vi "AutomatedTransfer_v2.vi"() -> ()   [LabVIEW 2013]
uses:
  controls/Control Configuration.ctl
  controls/Digital Controller.ctl
  controls/Motion Observer.ctl
  controls/UI Data.ctl
  controls/All FPGA Configuration Values.ctl
  controls/FPGA State.ctl
  controls/Raw Values.ctl
  Globals/Global - All UI Loop Stop.vi
  Globals/Global - UI Stream and Variable Connections.vi
  Globals/Global - Configuration Options.vi
  support/User Event - Stop/User Event - Stop.lvlib
  support/Message Queue/Message Queue.lvlib
  <vilib>/Analysis/NI_AALBase.lvlib
panel:
  in  "Switch to Safe State":bool
  in  "Exit":bool
  out "System Status":string="\n8/4/2014 6:26:47 PM: RT Error 91 - Variant To Data in RT Main.vi\n8/4/2014 6:26:32 PM: RT Error 91 - Variant To Data in RT Main.vi\n8/4/2014 6:26:21 PM: RT Error 91 - Variant To Data in RT Main.vi\n8/4/2014 6:26:03 PM: RT Error 91 - Variant To Data in RT Main.vi\n8/4/2014 6:25:47 PM: RT Error 91 - Variant To Data in RT Main.vi\n8/4/2014 6:25:36 PM: RT Error 91 - Variant To Data in RT Main.vi\n6/10/2014 3:19:43 PM: UI Error -1950679035 - Read Variable in AutomatedTransfer_v2.vi\n5/12/2014 3:31:58 PM: UI Error -314220 - Read Single Element from Stream in UI - Read Stream from RT.vi->UI Main.vi\n5/12/2014 3:31:58 PM: UI Error -314220 - Read Single Element from Stream in UI - Read Stream from RT.vi->UI Main.vi\n5/12/2014 3:31:58 PM: UI Error -314220 - Read Single Element from Stream in UI - Read Stream from RT.vi->UI Main.vi\n5/12/2014 3:31:58 PM: UI Error -314220 - Read Single Element from Stream in UI - Read Stream from RT.vi->UI Main.vi\n5/12/2014 3:31:58 PM: UI Error -314220 - Read Single Element from Stream in UI - Read Stream from RT.vi->UI Main.vi\n5/12/2014 3:31:58 PM: UI Error -314220 - Read Single Element from Stream in UI - Read Stream from RT.vi->UI Main.vi\n5/12/2014 3:31:58 PM: UI Error -314220 - Read Single Element from Stream in UI - Read Stream from RT.vi->UI Main.vi\n5/12/2014 3:31:58 PM: UI Error -314220 - Read Single Element from Stream in UI - Read Stream from RT.vi->UI Main.vi\n5/12/2014 3:31:58 PM: UI Error -314220 - Read Single Element from Stream in UI - Read Stream from RT.vi->UI Main.vi\n5/12/2014 3:31:58 PM: UI Error -314220 - Read Single Element from Stream in UI - Read Stream from RT.vi->UI Main.vi\n5/12/2014 3:31:58 PM: UI Error -314220 - Read Single Element from Stream in UI - Read Stream from RT.vi->UI Main.vi\n5/12/2014 3:31:58 PM: UI Error -314220 - Read Single Element from Stream in UI - Read Stream from RT.vi->UI Main.vi\n5/12/2014 3:31:58 PM: UI Error -314220 - Read Single Element from Stream in UI - Read Stream from RT.vi->UI Main.vi\n5/12/2014 3:31:58 PM: UI Error -314220 - Read Single Element from Stream in UI - Read Stream from RT.vi->UI Main.vi\n5/12/2014 3:31:58 PM: UI Error -314220 - Read Single Element from Stream in UI - Read Stream from RT.vi->UI Main.vi\n5/12/2014 3:31:58 PM: UI Error -314220 - Read Single Element from Stream in UI - Read Stream from RT.vi->UI Main.vi\n5/12/2014 3:31:58 PM: UI Error -314220 - Write Single Element to Stream in UI Main.vi\n5/12/2014 3:31:36 PM: UI Error -314004 - Create Network Stream Writer Endpoint in UI - Initiate Connection.vi->UI Main.vi\n5/6/2014 11:02:04 PM: UI Error -314220 - Write Single Element to Stream in UI Main.vi"
  out "Current FPGA Control Mode":u16(ring) items=["Safe State", "Manual", "Control (PID)"]
  in  "Settings Tab":T1(tab)
  out "Stage stop position (mm):":dbl=99.99983984375 format="%#.2g"
  out "Test LED":bool
  out "Roller LED":bool=TRUE
  in  "Test control":bool
  in  "Disable test control":bool
  in  "Stage speed (mm/s):":dbl=21.0 min=0.2 max=21.0
  out "Force results (N)":cluster{dbl[], dbl[]}(graph)
  in  "Save Results":bool
  in  "Stop Test":bool
  in  "Run Test":bool
  in  "Stop dwell time (s):":dbl=2.0 min=0.0
  in  "Start dwell time (s):":dbl=2.0 min=0.0
  in  "Travel distance (mm):":dbl=50.0 min=-150.0 max=150.0 step=0.1
  in  "Contact force (N):":fxp<+/-,20,7>=4.0
  out "Measured contact force (N):":dbl
  out "Stage position (mm):":dbl format="%#.2g"
  out "Fthresh (N):":fxp<+/-,16,8>=2.0 format="%.3g"
  in  "Home position (mm)":dbl=3.5
  in  "Stop roller":bool
  in  "Speed (mm/s):":dbl=2.0 min=0.2 max=5.0
  in  "Contact roller":bool
  in  "Disable roller control":bool
  in  "Roller control":bool
  in  "Home Roller":bool
  in  "Auto tare":bool=TRUE
  out "Position (mm):":dbl
  out "Force (N):":dbl
  out "Max speed (mm/s):":dbl=21.0
  out "Max position (mm):":dbl=151.49760546875
  in  "Position (mm):":dbl=85.0 min=0.0 max=150.0 step=0.1
  in  "Stage speed (mm/s):":dbl=21.0 min=0.2 max=21.0
  out "Stage position (mm):":dbl=99.9996015625 format="%#.2g"
  in  "Go stage":bool
  in  "Stop stage":bool
  in  "Home stage":bool
  out "path":path
  in  "Motion Observer":T2
  in  "Control period (ticks)":u32=40000
  in  "Find tare offset":bool=TRUE
  in  "Channel 3 Setpoint":fxp<+/-,16,5>
  in  "Channel 2 Setpoint":fxp<+/-,16,5>
  in  "Channel 1 Setpoint":fxp<+/-,20,7>=24.0
  in  "Channel 0 Setpoint":fxp<+/-,20,7>=4.0
  in  "Update Control Configuration":bool
  in  "Control Configurations":T3[](array[typedef])=[{"PID Gains"={"proportional gain (Kc)"=55.0, "integral gain (Kc*Ts/Ti)"=0.0, "derivative gain (Kc*Td/Ts)"=0.0}, "Output Range"={"output high"=50.0, "output low"=-50.0}}, {"PID Gains"={"proportional gain (Kc)"=0.0, "integral gain (Kc*Ts/Ti)"=0.0, "derivative gain (Kc*Td/Ts)"=0.0}, "Output Range"={"output high"=10.0, "output low"=-10.0}}, {"PID Gains"={"proportional gain (Kc)"=0.0, "integral gain (Kc*Ts/Ti)"=0.0, "derivative gain (Kc*Td/Ts)"=0.0}, "Output Range"={"output high"=10.0, "output low"=-10.0}}, {"PID Gains"={"proportional gain (Kc)"=0.0, "integral gain (Kc*Ts/Ti)"=0.0, "derivative gain (Kc*Td/Ts)"=0.0}, "Output Range"={"output high"=10.0, "output low"=-10.0}}]
  in  "Run Control":bool
  in  "Stop Control":bool
  in  "Digital Controller":T4
  out "Offset (N)":fxp<+/-,16,8>=0.16796875
  in  "Channel 3 Manual Value":fxp<+/-,16,5>
  in  "Channel 2 Manual Value":fxp<+/-,16,5>
  in  "Channel 1 Manual Value":fxp<+/-,16,5>
  in  "Channel 0 Manual Value":fxp<+/-,16,5>
  in  "Run Manual":bool
  in  "Stop Manual":bool
  in  "Retain data":bool
  out "F std":dbl=0.005665196330386121 format="%#_4g"
  out "F avg":dbl=-0.0348828125 format="%#_4g"
  in  "Clear Button":bool
  in  "Pause Button":bool
  in  "Save As Button":bool
  in  "Display frequency (Hz)":dbl=100.0 min=1.0 step=1.0
  out "Inputs (mV or V)":cluster{dbl[], dbl[]}[](graph)
  in  "Number of points":i32=500 min=1 max=999999999
  out "Force (N)":cluster{dbl[], dbl[]}(graph)
  out "V*":cluster{dbl[], dbl[]}(graph)
  out "Roller position (mm)":cluster{dbl[], dbl[]}(graph)
  out "Control loop frequency (Hz)":u32=4294967295
  out "Stage position (mm)":cluster{dbl[], dbl[]}(graph)
  out "Actual Loop Period (ticks)":u32
  out "Largest Contiguous Memory (bytes)":dbl(graph)
  out "CPU Usage (%)":dbl(graph)
  out "Connected?":bool=TRUE
  in  "Connect to Controller":bool
  in  "Controller Address":string="169.254.66.100"
  # "LabVIEW FPGA Control on CompactRIO"
  # "Connection Settings"
  # "Roller panel"
  # "Stage panel"
  # "To do: \n-Wire appropriate connections into R2R-Controller\n-Update Monitoring Loop Rate by changing Display Rate \n  Note: with 1 ms rate, the program hangs\n-Clean up noise in load cell when V* acts"
  # "Warning: Home cannot be stopped"
  # "Test panel"
  # "Force Command (N)"
  # "Position Command (mm)"
  # "Current Command (Testing)"
  # "Control period and setpoint changes are sent to the target automatically."
  # "Control Configuration changes are sent to the target when you click \"Update Control Configurations\"."
  # "Not used"
  # "Not used"
  # "Not used"
  # "F ="
  # "+/-"
  # "N"
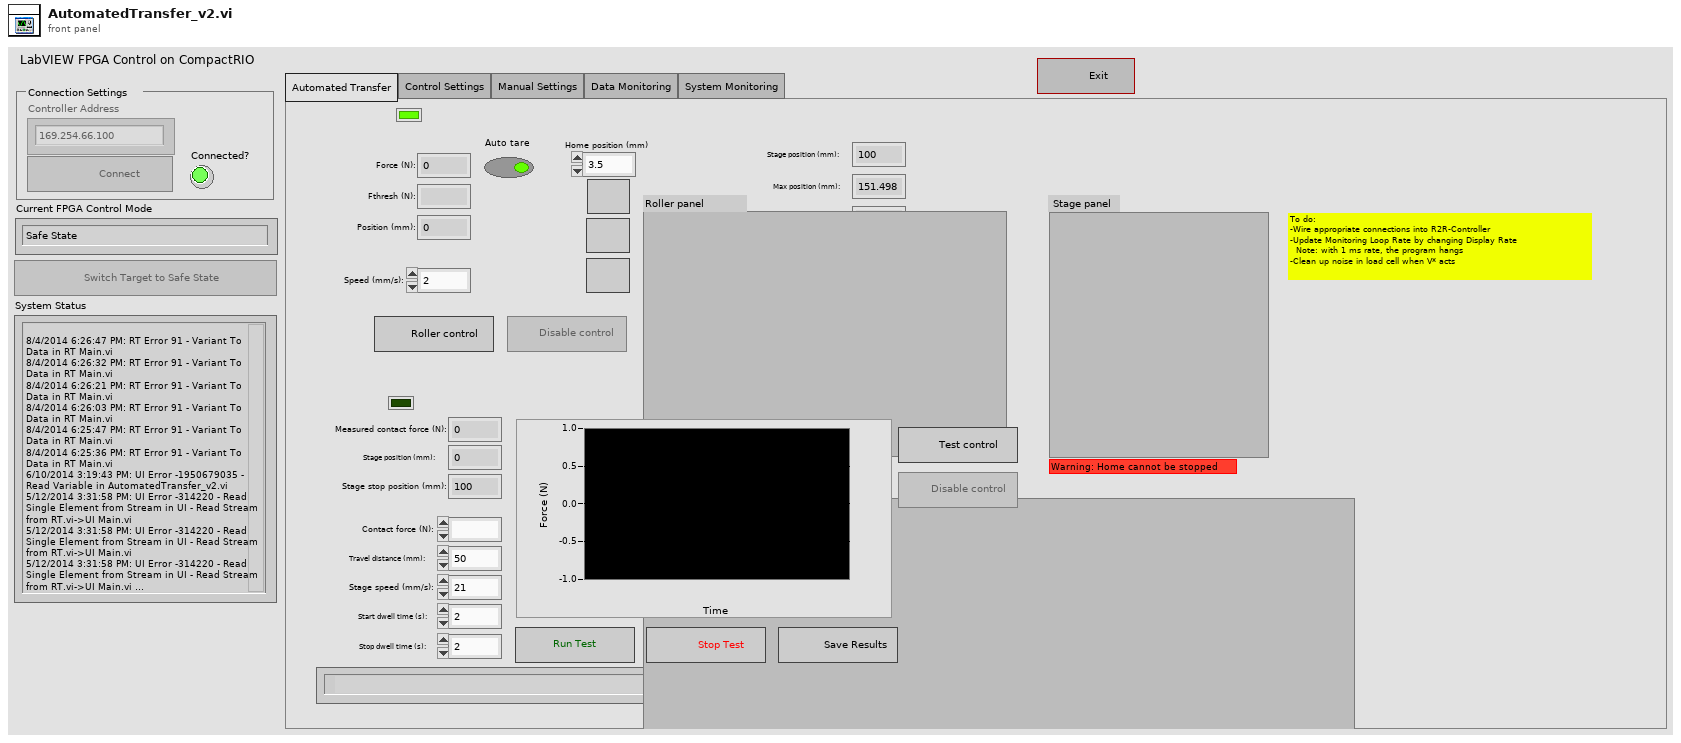
[diagram p1: front panel]
types:
  T1 = enum32{"Automated Transfer", "Control Settings", "Manual Settings", "Data Monitoring", "System Monitoring"}
  T2 = typedef "Motion Observer.ctl" = cluster{"bo (kg/s)":fxp<+/-,20,7>, "kso (N/m)":fxp<+/-,20,7>, "kiso (N/m)":fxp<+/-,20,7>}
  T3 = typedef "Control Configuration.ctl" = cluster{"PID Gains":cluster{"proportional gain (Kc)":fxp<+/-,16,8>, "integral gain (Kc*Ts/Ti)":fxp<+/-,16,8>, "derivative gain (Kc*Td/Ts)":fxp<+/-,16,8>}, "Output Range":cluster{"output high":fxp<+/-,16,7>, "output low":fxp<+/-,16,7>}}
  T4 = typedef "Digital Controller.ctl" = cluster{"kvc (N/m)":fxp<+,16,12>, "ymod (-)":fxp<+/-,16,5>, "Mar (kg)":fxp<+/-,16,8>, "Foff (N)":fxp<+/-,16,8>, "Fthresh (N)":fxp<+/-,16,5>, "ba (kg/s)":fxp<+/-,16,5>, "ksa (N/m)":fxp<+/-,16,5>, "kisa (N/m)":fxp<+/-,16,5>, "k_backemf":fxp<+/-,16,5>, "Frr (N/s)":fxp<+/-,16,5>, "xrr (mm/s)":fxp<+/-,16,5>, "bp (kg/s)":fxp<+/-,16,5>, "k_1 (1/s)":fxp<+/-,16,5>, "k_2 (1/s)":fxp<+/-,16,5>}
  T5 = typedef "UI Data.ctl" = cluster{"Switch to Safe State Ref":refnum<vi>, "Run Manual Ref":refnum<vi>, "Stop Manual Ref":refnum<vi>, "Run Control Ref":refnum<vi>, "Stop Control Ref":refnum<vi>, "Update Control Configurations Ref":refnum<vi>, "Ch 0 Setpoint Ref":refnum<vi>, "Ch 1 Setpoint Ref":refnum<vi>, "Ch 2 Setpoint Ref":refnum<vi>, "Ch 3 Setpoint Ref":refnum<vi>, "Ch 0 Manual Ref":refnum<vi>, "Ch 1 Manual Ref":refnum<vi>, "Ch 2 Manual Ref":refnum<vi>, "Ch 3 Manual Ref":refnum<vi>, "Control Configurations Ref":refnum<vi>, "Control period (ticks) Ref":refnum<vi>, "Roller control":refnum<vi>, "Disable roller control":refnum<vi>, "Test control":refnum<vi>, "Disable test control":refnum<vi>, "Motion Observer":refnum<vi>, "Digital Controller":refnum<vi>}
  T6 = typedef "Message Queue.lvlib/All Message Queues.ctl" = cluster{"UI":refnum<queue>}
  T7 = enum16{"open", "replace", "create", "open or create", "replace or create", "replace or create with confirmation"}
  T8 = cluster{"Channel 0 Setpoint":fxp<+/-,20,7>, "Channel 1 Setpoint":fxp<+/-,20,7>, "Channel 2 Setpoint":fxp<+/-,16,5>, "Channel 3 Setpoint":fxp<+/-,16,5>}
  T9 = cluster{"Channel 0 Manual Value":fxp<+/-,16,5>, "Channel 1 Manual Value":fxp<+/-,16,5>, "Channel 2 Manual Value":fxp<+/-,16,5>, "Channel 3 Manual Value":fxp<+/-,16,5>}
  T10 = typedef "Variable References.ctl" = cluster{"CPU Usage":refnum<k21>, "Contiguous Memory":refnum<k21>, "Input Values":refnum<k21>, "Output Values":refnum<k21>, "FPGA Mode":refnum<k21>, "Actual Loop Period":refnum<k21>}
  T11 = typedef "Raw Values.ctl" = cluster{"Channel 0":fxp<+/-,20,7>, "Channel 1":fxp<+/-,20,7>, "Channel 2":fxp<+/-,20,7>, "Channel 3":fxp<+/-,20,14>}
  T12 = cluster{"Channel 0":dbl, "Channel 1":dbl, "Channel 2":dbl, "Channel 3":dbl}
  T13 = cluster{fxp<+/-,16,5>, "Channel 1 Manual Value":fxp<+/-,16,5>, "Channel 2 Manual Value":fxp<+/-,16,5>, "Channel 3 Manual Value":fxp<+/-,16,5>}
  T14 = cluster{"fixed-point type":fxp<+/-,16,5>, "Channel 1 Manual Value":fxp<+/-,16,5>, "Channel 2 Manual Value":fxp<+/-,16,5>, "Channel 3 Manual Value":fxp<+/-,16,5>}
  T15 = cluster{"Contact force (N): ":fxp<+/-,20,7>, "Channel 1 Setpoint":fxp<+/-,20,7>, "Channel 2 Setpoint":fxp<+/-,16,5>, "Channel 3 Setpoint":fxp<+/-,16,5>}
  T16 = cluster{"Message":string, "Message Data":variant}
  T17 = typedef "All FPGA Configuration Values.ctl" = cluster{"FPGA State":T18, "Manual Values":T11, "Setpoints":T11, "Control Configurations":T3[]}
  T18 = typedef "FPGA State.ctl" = enum16{"Safe State", "Manual", "Control (PID)"}
  T19 = cluster{"Digital Controller":T4, "Motion Observer":T2}
  T20 = cluster{string, cluster{"Digital Controller":T4, "Motion Observer":T2}}
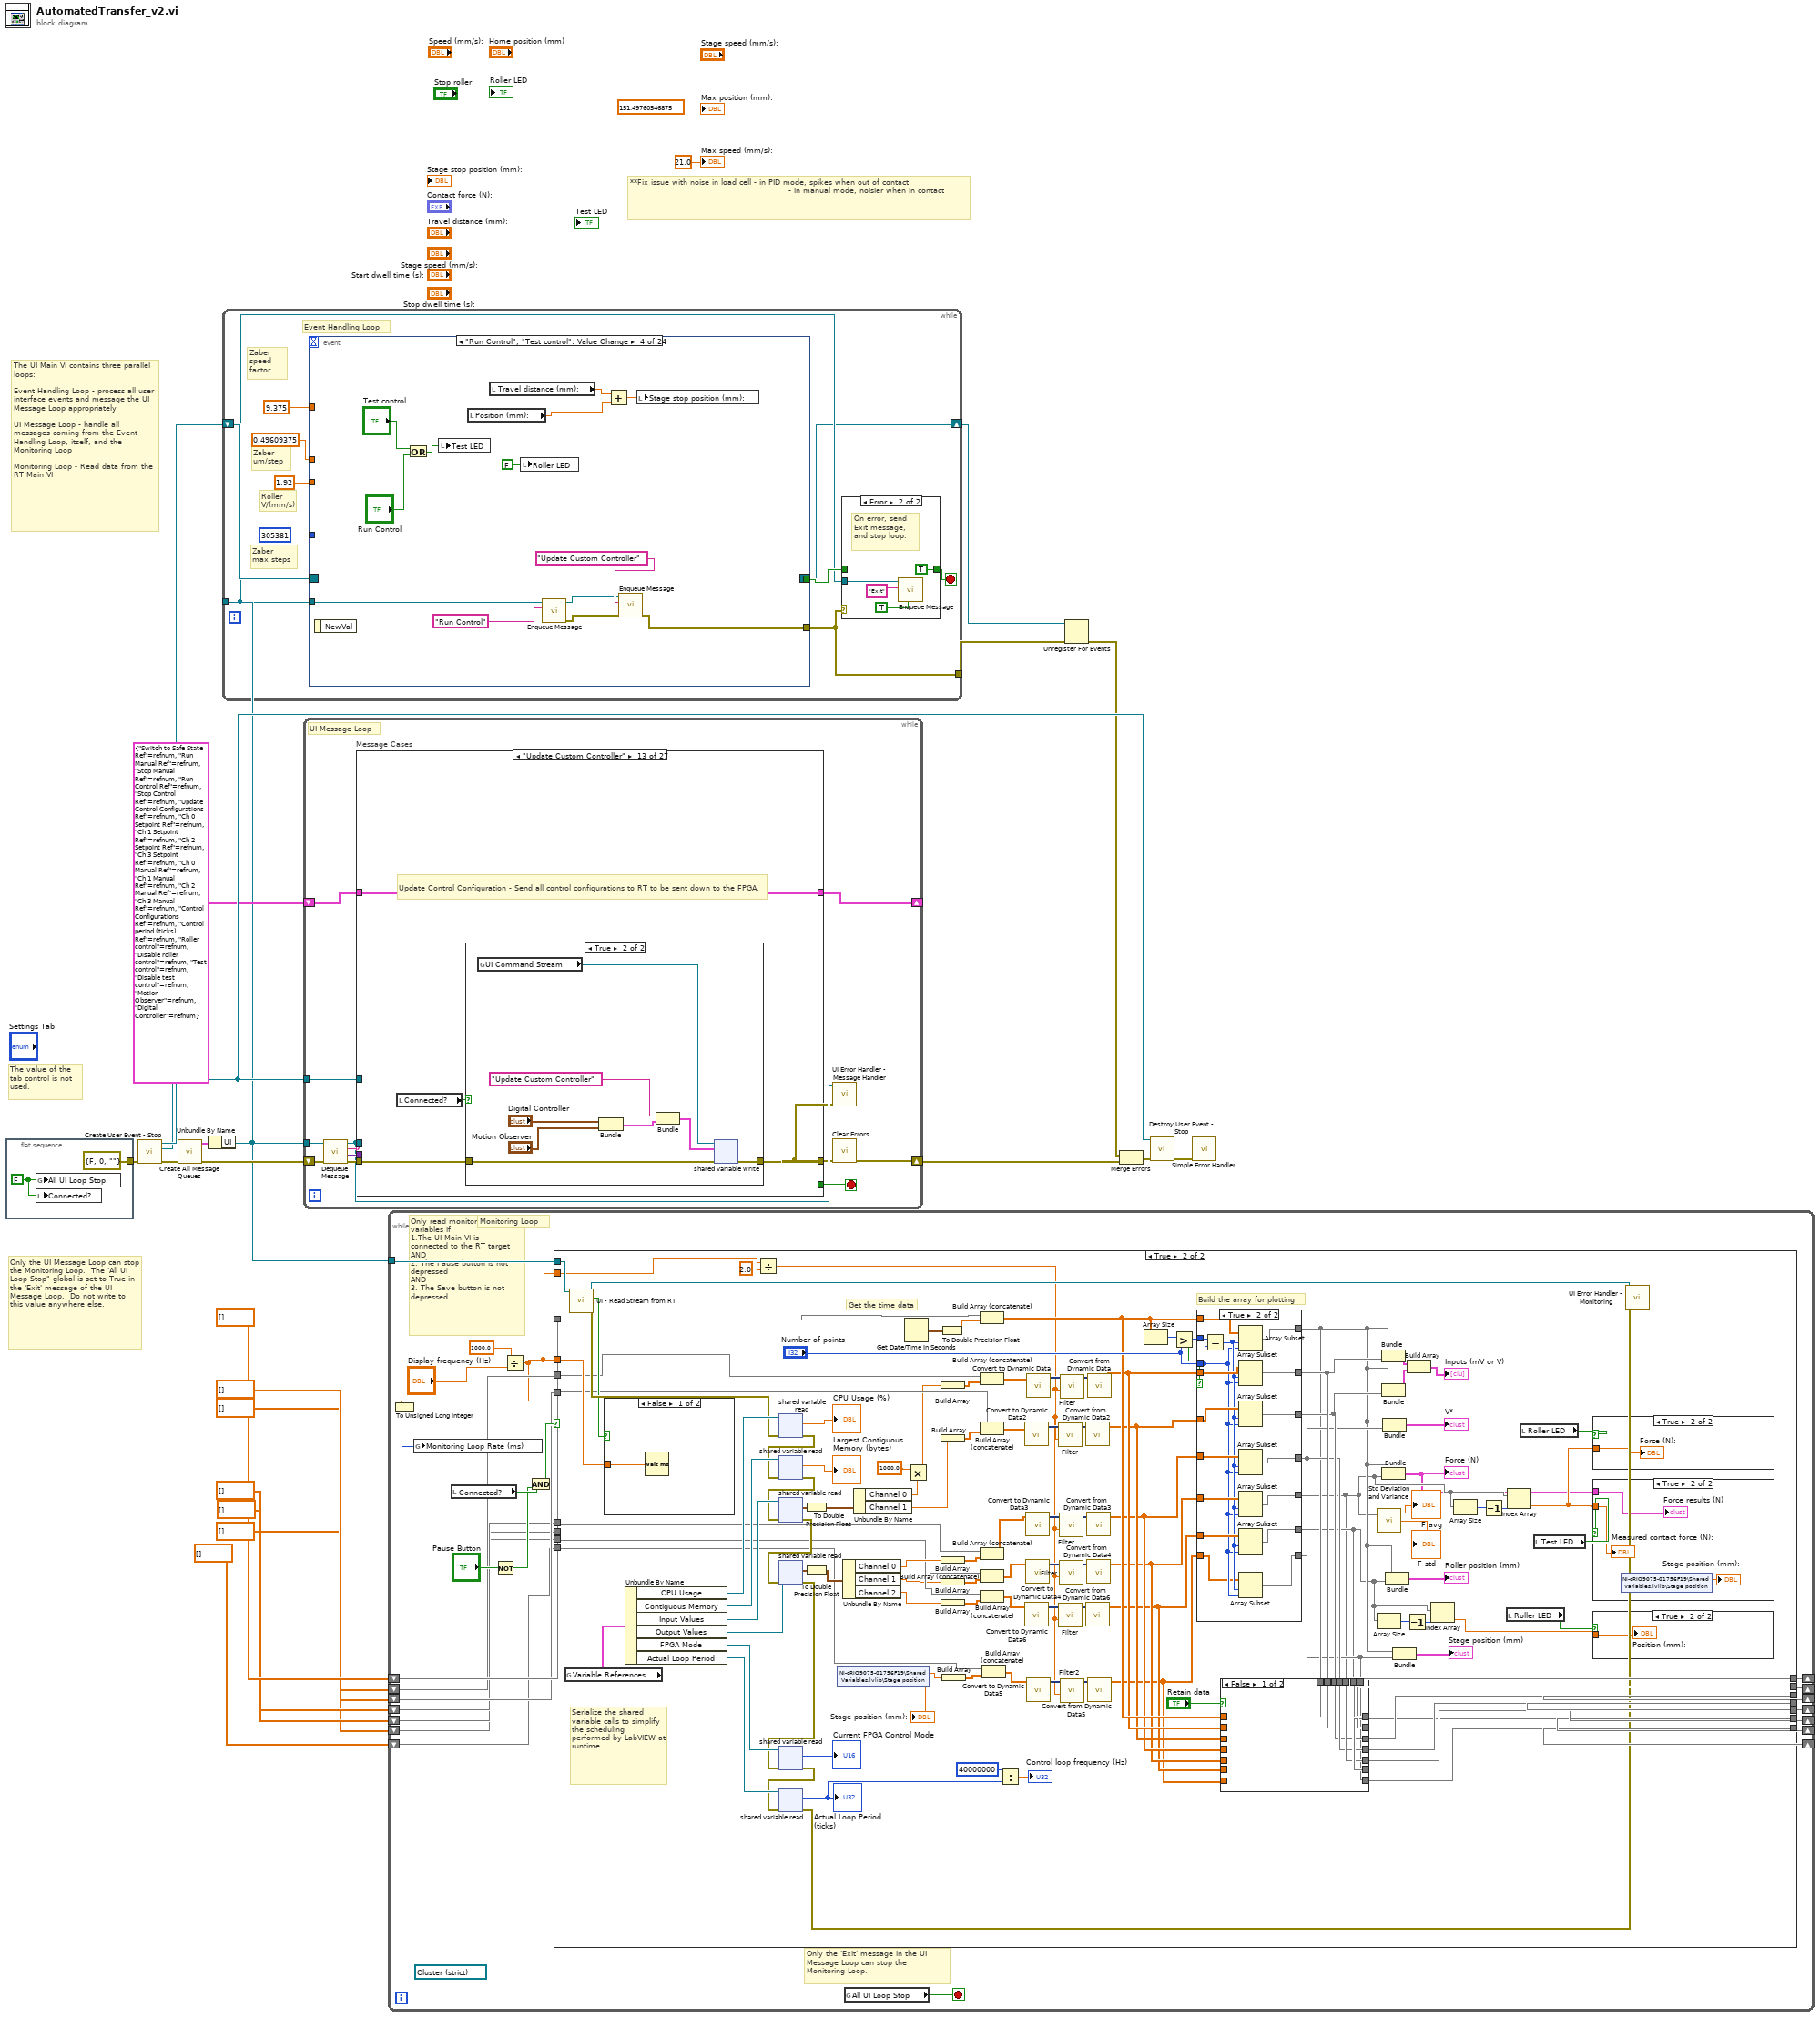
[diagram p0: block diagram]
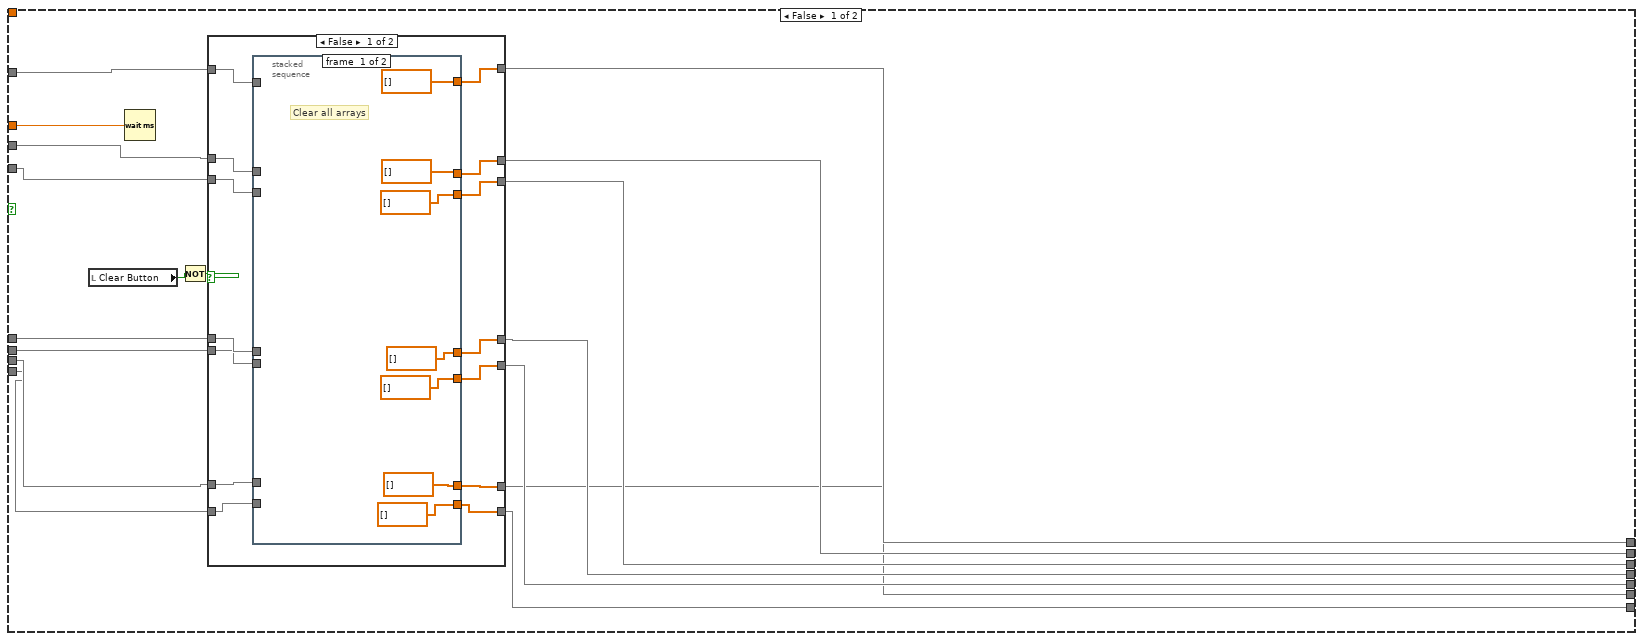
[diagram p2: hidden frame]
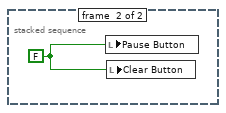
[diagram p3: hidden frame]
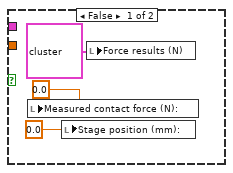
[diagram p5: hidden frame]
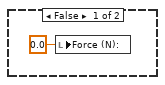
[diagram p6: hidden frame]
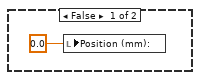
[diagram p7: hidden frame]
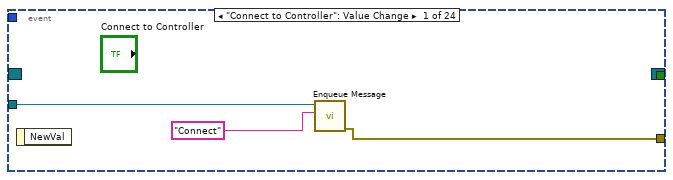
[diagram p12: hidden frame]
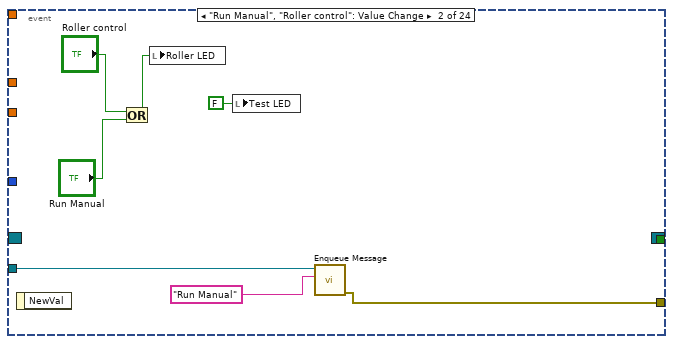
[diagram p13: hidden frame]
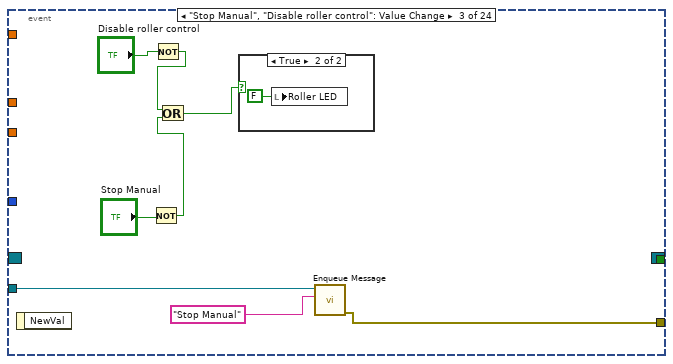
[diagram p14: hidden frame]
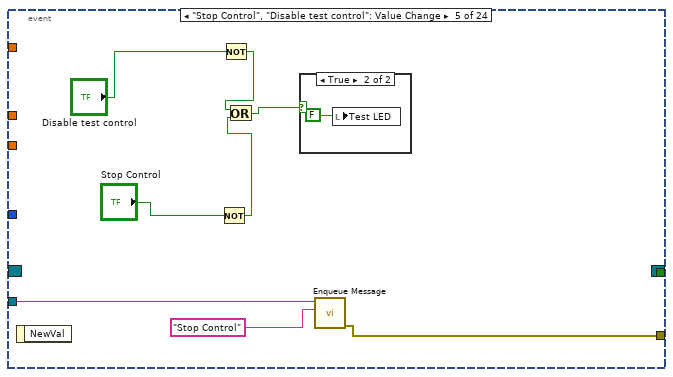
[diagram p16: hidden frame]
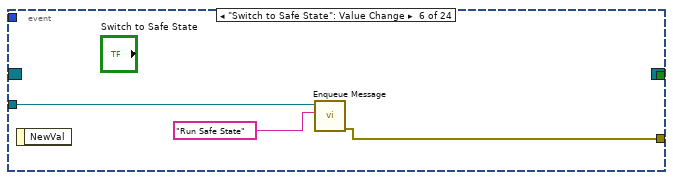
[diagram p18: hidden frame]
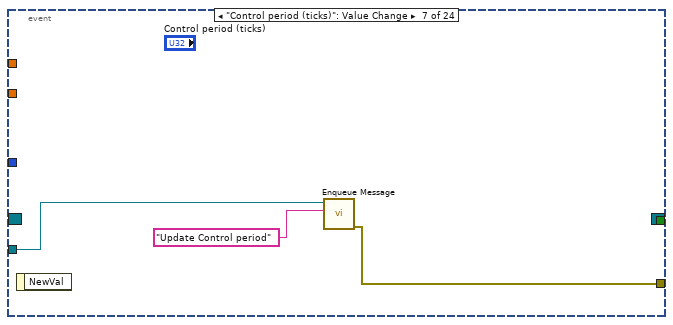
[diagram p19: hidden frame]
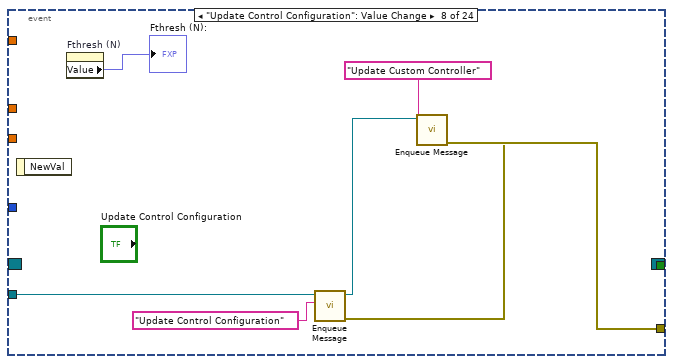
[diagram p20: hidden frame]
diagram:
  # "**Fix issue with noise in load cell - in PID mode, spikes when out of contact\n                                                          - in manual mode, noisier when in contact"
  # "The UI Main VI contains three parallel loops:\n\nEvent Handling Loop - process all user interface events and message the UI Message Loop appropriately\n\nUI Message Loop - handle all messages coming from the Event Handling Loop, itself, and the Monitoring Loop\n\nMonitoring Loop - Read data from the RT Main VI"
  # "The value of the tab control is not used."
  # "Only the UI Message Loop can stop the Monitoring Loop.  The 'All UI Loop Stop\" global is set to True in the 'Exit' message of the UI Message Loop.  Do not write to this value anywhere else."
  n1 = flat-sequence {
    tunnel: [errorcluster {"status"=FALSE, "code"=0, "source"=""} ("error in (no error)")] -> w10
    frame #0 {
      w24 = FALSE
      n2 = global write "Global - All UI Loop Stop.vi" "All UI Loop Stop"(w24) -> ()
      n3 = local write "Connected?"(w24) -> ()
    }
  }
  n4 = call "Create User Event - Stop.vi"("error in (no error)"=w10) -> ("error out"=w18:errorcluster, "User Event - Stop"=w19:refnum<user-event>, "Stop Event Registration Refnum"=w20:refnum<event-registration>)  [unwired: 8 in]
  n5 = call "Create All Message Queues.vi"("error in (no error)"=w18) -> ("error out"=w16:errorcluster, "Message Queues out"=w17:T6)  [unwired: 9 in]
  n6 = Unbundle By Name(w17) -> ("UI"=w11:refnum<queue>)
  n7 = while {
    tunnel: w11 -> [w31]
    tunnel: [w33] -> w22
    shift-right: [w30] -> w14
    shift-left: w20 -> [w32]
    stop <- w34 stop-if-true
    # "Zaber \nmax steps"
    # "Zaber \nspeed factor"
    # "Zaber \num/step"
    # "Roller \nV/(mm/s)"
    # "Event Handling Loop"
    n8 = event shown="[3] \"Run Control\", \"Test control\": Value Change" {
      selector: w32 -> [_ _ _ _ _ _ _ _ _ _ _ _ _ _ _ _ _ _ _ _ _ _ _ _]
      dyn-events: [_ _ _ _ _ _ _ _ _ _ _ _ _ _ _ _ _ _ _ _ _ _ _ _] -> w30
      timeout: _ -> [_ _ _ _ _ _ _ _ _ _ _ _ _ _ _ _ _ _ _ _ _ _ _ _]
      tunnel: [_ _ _ _ _ _ _ _ _ _ _ _ _ _ _ _ _ _ _ _ _ TRUE ("Discard?") _ _] -> w35
      tunnel: w31 -> [w41 w48 w56 w71 w78 w82 w87 w94 w97 w106 w113 w138 w143 w174 w207 w218 w225 w269 w276 _ w295 _ _ _]
      tunnel: [w43 w50 w58 w67 w80 w84 w85 w91 w96 w105 w112 w141 w142 w173 w206 w219 w224 w268 w274 _ _ _ _ _] -> w33
      tunnel: 1.92 -> [_ _ _ _ _ _ _ _ _ _ _ _ _ w172 _ _ _ _ _ _ w294 _ _ _]
      tunnel: 0.49609375 -> [_ _ _ _ _ _ _ _ _ _ _ _ _ _ _ _ w223 _ _ _ w293 _ _ _]
      tunnel: 9.375 -> [_ _ _ _ _ _ _ _ _ _ _ _ _ _ _ _ w222 _ _ _ w292 _ _ _]
      tunnel: 305381 -> [_ _ _ _ _ _ _ _ _ _ _ _ _ _ _ _ w221 _ _ _ w291 _ _ _]
      event "Connect to Controller": Value Change {
        n9 = event-data() -> ()  [unwired: 1 in, 1 out]
        n10 = call "Enqueue Message.vi"("Message"="Connect", "Message Queue"=w41) -> ("error out"=w43:errorcluster)  [unwired: 8 in, 1 out]
      }
      event "Run Manual", "Roller control": Value Change {
        n11 = event-data() -> ()  [unwired: 1 in, 1 out]
        n12 = Or(x="Roller control", y="Run Manual") -> (x .or. y?=w45:bool)
        n13 = local write "Roller LED"(w45) -> ()
        n14 = local write "Test LED"(FALSE ("Test LED")) -> ()
        n15 = call "Enqueue Message.vi"("Message"="Run Manual", "Message Queue"=w48) -> ("error out"=w50:errorcluster)  [unwired: 8 in, 1 out]
      }
      event "Stop Manual", "Disable roller control": Value Change {
        n16 = event-data() -> ()  [unwired: 1 in, 1 out]
        n17 = Not(x="Stop Manual") -> (.not. x?=w53:bool)
        n18 = Not(x="Disable roller control") -> (.not. x?=w52:bool)
        n19 = Or(x=w52, y=w53) -> (x .or. y?=w51:bool)
        n20 = case shown="True" w51 {
          frame False {
          }
          frame True {
            n21 = local write "Roller LED"(FALSE) -> ()
          }
        }
        n22 = call "Enqueue Message.vi"("Message"="Stop Manual", "Message Queue"=w56) -> ("error out"=w58:errorcluster)  [unwired: 8 in, 1 out]
      }
      event "Run Control", "Test control": Value Change {
        n23 = event-data() -> ()  [unwired: 1 in, 1 out]
        n24 = Or(x="Test control", y="Run Control") -> (x .or. y?=w64:bool)
        n25 = local write "Test LED"(w64) -> ()
        n26 = local read "Position (mm):"() -> (w62:dbl)
        n27 = local read "Travel distance (mm):"() -> (w61:dbl)
        n28 = local write "Roller LED"(FALSE ("Roller LED")) -> ()
        n29 = call "Enqueue Message.vi"("Message"="Run Control", "Message Queue"=w71) -> ("error out"=w68:errorcluster, "dup Message Queue"=w69:refnum<queue>)  [unwired: 8 in]
        n30 = Add(x=w61, y=w62) -> (x+y=w60:dbl)
        n31 = call "Enqueue Message.vi"("error in (no error)"=w68, "Message"="Update Custom Controller", "Message Queue"=w69) -> ("error out"=w67:errorcluster)  [unwired: 7 in, 1 out]
        n32 = local write "Stage stop position (mm):"(w60) -> ()
      }
      event "Stop Control", "Disable test control": Value Change {
        n33 = event-data() -> ()  [unwired: 1 in, 1 out]
        n34 = Not(x="Stop Control") -> (.not. x?=w74:bool)
        n35 = Not(x="Disable test control") -> (.not. x?=w75:bool)
        n36 = Or(x=w75, y=w74) -> (x .or. y?=w73:bool)
        n37 = case shown="True" w73 {
          frame False {
          }
          frame True {
            n38 = local write "Test LED"(FALSE) -> ()
          }
        }
        n39 = call "Enqueue Message.vi"("Message"="Stop Control", "Message Queue"=w78) -> ("error out"=w80:errorcluster)  [unwired: 8 in, 1 out]
      }
      event "Switch to Safe State": Value Change {
        n40 = event-data() -> ()  [unwired: 1 in, 1 out]
        n41 = call "Enqueue Message.vi"("Message"="Run Safe State", "Message Queue"=w82) -> ("error out"=w84:errorcluster)  [unwired: 8 in, 1 out]
      }
      event "Control period (ticks)": Value Change {
        n42 = event-data() -> ()  [unwired: 1 in, 1 out]
        n43 = call "Enqueue Message.vi"("Message"="Update Control period", "Message Queue"=w87) -> ("error out"=w85:errorcluster)  [unwired: 8 in, 1 out]
      }
      event "Update Control Configuration": Value Change {
        n44 = event-data() -> ()  [unwired: 1 in, 1 out]
        n45 = property on="Fthresh (N)" class="DigNum (strict)"() -> ("Value"=→"Fthresh (N):":fxp<+/-,16,5>)  [unwired: 2 in, 2 out]
        n46 = call "Enqueue Message.vi"("Message"="Update Control Configuration", "Message Queue"=w94) -> ("error out"=w89:errorcluster, "dup Message Queue"=w90:refnum<queue>)  [unwired: 8 in]
        n47 = call "Enqueue Message.vi"("error in (no error)"=w89, "Message"="Update Custom Controller", "Message Queue"=w90) -> ("error out"=w91:errorcluster)  [unwired: 7 in, 1 out]
      }
      event "Channel 0 Setpoint", "Channel 1 Setpoint", "Channel 2 Setpoint", "Channel 3 Setpoint": Value Change {
        n48 = event-data() -> ()  [unwired: 1 in, 1 out]
        n49 = Bundle("Channel 0 Setpoint"="Channel 0 Setpoint", "Channel 1 Setpoint"="Channel 1 Setpoint", "Channel 2 Setpoint"="Channel 2 Setpoint", "Channel 3 Setpoint"="Channel 3 Setpoint") -> (w95:T8)  [unwired: 1 in]
        n50 = call "Enqueue Message.vi"("Message Data"=w95, "Message"="Update Setpoints", "Message Queue"=w97) -> ("error out"=w96:errorcluster)  [unwired: 7 in, 1 out]
      }
      event "Channel 0 Manual Value", "Channel 1 Manual Value", "Channel 2 Manual Value", "Channel 3 Manual Value": Value Change {
        n51 = event-data() -> ()  [unwired: 1 in, 1 out]
        n52 = Bundle("Channel 0 Manual Value"="Channel 0 Manual Value", "Channel 1 Manual Value"="Channel 1 Manual Value", "Channel 2 Manual Value"="Channel 2 Manual Value", "Channel 3 Manual Value"="Channel 3 Manual Value") -> (w103:T9)  [unwired: 1 in]
        n53 = call "Enqueue Message.vi"("Message Data"=w103, "Message"="Update Manual Values", "Message Queue"=w106) -> ("error out"=w105:errorcluster)  [unwired: 7 in, 1 out]
      }
      event "Find tare offset", "Auto tare": Value Change {
        (unwired) fxp<+/-,16,8> 0.0 ("Value")
        # "When Auto tare is pressed, the offset force (N) is calculated. This value is automaticaly \ninputted into the Offset weight control of Other Controller Gains."
        n54 = event-data() -> ()  [unwired: 1 in, 1 out]
        n55 = Or(x="Find tare offset", y="Auto tare") -> (x .or. y?=w114:bool)
        n56 = stacked-sequence {
          tunnel: 400 -> [w119 w132 _ _]
          tunnel: w114 -> [w118 _ _ _]
          tunnel: w113 -> [_ _ _ w136]
          tunnel: [_ _ _ w135] -> w112
          frame #0 {
            n57 = case shown="True" w118 {
              tunnel: w119 -> [_ w121]
              frame False {
                n58 = local write "Offset (N)"(0.0 ("Test")) -> ()
              }
              frame True {
                n59 = for {
                  N: w121 -> [_]
                  n60 = global read "Global - UI Stream and Variable Connections.vi" "Variable References"() -> (w125:T10)
                  n61 = Unbundle By Name(w125) -> ("Output Values"=w126:refnum<k21>)
                  n62 = shared-variable-read(w126) -> (w127:T11)  [unwired: 1 in, 3 out]
                  n63 = local read "Offset (N)"() -> (w124:fxp<+/-,16,8>)
                  n64 = To Double Precision Float(number=w127) -> (double precision float=w128:T12)
                  n65 = Unbundle(w128) -> ("Channel 1"=w122:dbl)  [unwired: 3 out]
                  n66 = Add(x=w122, y=w124) -> (x+y=w123:dbl)
                  n67 = local write "Offset (N)"(w123) -> ()
                  n68 = Wait (ms)(milliseconds to wait=u32 5) -> ()  [unwired: 1 out]
                }
              }
            }
          }
          frame #1 {
            n69 = local read "Offset (N)"() -> (w133:fxp<+/-,16,8>)
            n70 = To Double Precision Float(number=w132) -> (double precision float=w131:dbl)
            n71 = Divide(x=w133, y=w131) -> (x/y=w130:dbl)
            n72 = local write "Offset (N)"(w130) -> ()
          }
          frame #2 {
            n73 = local read "Offset (N)"() -> (w134:fxp<+/-,16,8>)
            n74 = property on="Foff (N)" class="DigNum (strict)"("Value"=w134) -> ()  [unwired: 2 in, 2 out]
          }
          frame #3 {
            n75 = call "Enqueue Message.vi"("Message"="Update Custom Controller", "Message Queue"=w136) -> ("error out"=w135:errorcluster)  [unwired: 8 in, 1 out]
          }
        }
        "Offset (N)" <- 0.0 ("Offset weight (N)")
      }
      event "Exit": Value Change {
        w139 = TRUE  # Priority Message
        # "The UI Message Loop handles sending the Exit message to other loops."
        n76 = event-data() -> ()  [unwired: 1 in, 1 out]
        n77 = call "Enqueue Message.vi"("Priority Message? (F)"=w139, "Message"="Exit", "Message Queue"=w138) -> ("error out"=w141:errorcluster)  [unwired: 7 in, 1 out]
      }
      event "Home Roller": Value Change {
        n78 = event-data() -> ()  [unwired: 1 in, 1 out]
        n79 = for {
          N: 3 -> [_]
          tunnel: w143 -> [w146]
          tunnel: [w145] -> w142
          i -> [w147]
          n80 = case shown="2" w147 {
            tunnel: w146 -> [_ w149 _ w169]
            tunnel: [_ w148 _ w168] -> w145
            frame Default {
            }
            frame 0 {
              # "V/(mm/s)"
              n81 = local read "Speed (mm/s):"() -> (w151:dbl)
              n82 = local read "Channel 1 Manual Value"() -> (w156:fxp<+/-,16,5>)
              n83 = local read "Channel 2 Manual Value"() -> (w155:fxp<+/-,16,5>)
              n84 = local read "Channel 3 Manual Value"() -> (w154:fxp<+/-,16,5>)
              n85 = Multiply(x=w151, y=-1.92) -> (x*y=w153:dbl)
              n86 = To Fixed-Point(number=w153) -> (fixed-point=w150:fxp<+/-,16,5>)  [unwired: 1 in]
              n87 = local write "Channel 0 Manual Value"(w150) -> ()
              n88 = Bundle(w150, "Channel 1 Manual Value"=w156, "Channel 2 Manual Value"=w155, "Channel 3 Manual Value"=w154) -> (w157:T13)  [unwired: 1 in]
              n89 = call "Enqueue Message.vi"("Message Data"=w157, "Message"="Home roller", "Message Queue"=w149) -> ("error out"=w148:errorcluster)  [unwired: 7 in, 1 out]
            }
            frame 1 {
              n90 = while {
                stop <- w162 stop-if-true
                n91 = local read "Home position (mm)"() -> (w159:dbl)
                n92 = local read "Position (mm):"() -> (w160:dbl)
                n93 = local read "Stop roller"() -> (w161:bool)
                n94 = Less?(x=w160, y=w159) -> (x < y?=w163:bool)
                n95 = Or(x=w163, y=w161) -> (x .or. y?=w162:bool)
              }
            }
            frame 2 {
              w167 = fxp<+/-,16,5> 0.0 ("fixed-point type")
              n96 = local read "Channel 3 Manual Value"() -> (w164:fxp<+/-,16,5>)
              n97 = local read "Channel 2 Manual Value"() -> (w165:fxp<+/-,16,5>)
              n98 = local read "Channel 1 Manual Value"() -> (w166:fxp<+/-,16,5>)
              n99 = local write "Channel 0 Manual Value"(w167) -> ()
              n100 = Bundle("fixed-point type"=w167, "Channel 1 Manual Value"=w166, "Channel 2 Manual Value"=w165, "Channel 3 Manual Value"=w164) -> (w170:T14)  [unwired: 1 in]
              n101 = call "Enqueue Message.vi"("Message Data"=w170, "Message"="Contact roller", "Message Queue"=w169) -> ("error out"=w168:errorcluster)  [unwired: 7 in, 1 out]
            }
          }
        }
      }
      event "Contact roller": Value Change {
        n102 = event-data() -> ()  [unwired: 1 in, 1 out]
        n103 = for {
          N: 3 -> [_]
          tunnel: w174 -> [w178]
          tunnel: [w177] -> w173
          tunnel: w172 -> [w176]
          i -> [w179]
          n104 = case shown="1" w179 {
            tunnel: w178 -> [_ w182 _ w198]
            tunnel: [_ w181 _ w197] -> w177
            tunnel: w176 -> [_ w180 _ _]
            frame Default {
            }
            frame 0 {
              n105 = local read "Speed (mm/s):"() -> (w187:dbl)
              n106 = local read "Channel 3 Manual Value"() -> (w183:fxp<+/-,16,5>)
              n107 = local read "Channel 1 Manual Value"() -> (w185:fxp<+/-,16,5>)
              n108 = local read "Channel 2 Manual Value"() -> (w184:fxp<+/-,16,5>)
              n109 = Multiply(x=w187, y=w180) -> (x*y=w188:dbl)
              n110 = To Fixed-Point(number=w188) -> (fixed-point=w186:fxp<+/-,16,5>)  [unwired: 1 in]
              n111 = local write "Channel 0 Manual Value"(w186) -> ()
              n112 = Bundle(w186, "Channel 1 Manual Value"=w185, "Channel 2 Manual Value"=w184, "Channel 3 Manual Value"=w183) -> (w189:T13)  [unwired: 1 in]
              n113 = call "Enqueue Message.vi"("Message Data"=w189, "Message"="Contact roller", "Message Queue"=w182) -> ("error out"=w181:errorcluster)  [unwired: 7 in, 1 out]
            }
            frame 1 {
              n114 = while {
                stop <- w193 stop-if-true
                n115 = local read "Fthresh (N):"() -> (w191:fxp<+/-,16,8>)
                n116 = local read "Force (N):"() -> (w196:dbl)
                n117 = local read "Stop roller"() -> (w194:bool)
                n118 = To Double Precision Float(number=w191) -> (double precision float=w192:dbl)
                n119 = Greater?(x=w196, y=w192) -> (0:w195:bool)
                n120 = Or(x=w195, y=w194) -> (x .or. y?=w193:bool)
              }
            }
            frame 2 {
              w199 = fxp<+/-,16,5> 0.0 ("fixed-point type")
              n121 = local read "Channel 1 Manual Value"() -> (w202:fxp<+/-,16,5>)
              n122 = local read "Channel 2 Manual Value"() -> (w201:fxp<+/-,16,5>)
              n123 = local read "Channel 3 Manual Value"() -> (w200:fxp<+/-,16,5>)
              n124 = local write "Channel 0 Manual Value"(w199) -> ()
              n125 = Bundle("fixed-point type"=w199, "Channel 1 Manual Value"=w202, "Channel 2 Manual Value"=w201, "Channel 3 Manual Value"=w200) -> (w203:T14)  [unwired: 1 in]
              n126 = call "Enqueue Message.vi"("Message Data"=w203, "Message"="Contact roller", "Message Queue"=w198) -> ("error out"=w197:errorcluster)  [unwired: 7 in, 1 out]
            }
          }
        }
      }
      event "Stop roller": Value Change {
        n127 = event-data() -> ()  [unwired: 1 in, 1 out]
        n128 = local read "Channel 2 Manual Value"() -> (w209:fxp<+/-,16,5>)
        n129 = local read "Channel 1 Manual Value"() -> (w210:fxp<+/-,16,5>)
        n130 = local read "Channel 3 Manual Value"() -> (w208:fxp<+/-,16,5>)
        n131 = Bundle("fixed-point type"=fxp<+/-,16,5> 0.0, "Channel 1 Manual Value"=w210, "Channel 2 Manual Value"=w209, "Channel 3 Manual Value"=w208) -> (w212:T14)  [unwired: 1 in]
        n132 = call "Enqueue Message.vi"("Message Data"=w212, "Message"="Stop roller", "Message Queue"=w207) -> ("error out"=w206:errorcluster)  [unwired: 7 in, 1 out]
      }
      event "Home stage": Value Change {
        n133 = event-data() -> ()  [unwired: 1 in, 1 out]
        n134 = Bundle(1, 1, 0, 1) -> (w213:cluster{i32, i32, i32, i32})  [unwired: 1 in]
        n135 = call "Enqueue Message.vi"("Message Data"=w213, "Message"="Home stage", "Message Queue"=w218) -> ("error out"=w219:errorcluster)  [unwired: 7 in, 1 out]
      }
      event "Go stage": Value Change {
        n136 = event-data() -> ()  [unwired: 1 in, 1 out]
        n137 = for {
          N: 2 -> [_]
          tunnel: w225 -> [w231]
          tunnel: [w230] -> w224
          tunnel: w223 -> [w229]
          tunnel: w222 -> [w228]
          tunnel: w221 -> [w227]
          i -> [w232]
          n138 = case shown="1" w232 {
            tunnel: w231 -> [_ w247 w260]
            tunnel: [_ w246 w259] -> w230
            tunnel: w229 -> [_ w234 _]
            tunnel: w228 -> [_ w233 _]
            tunnel: w227 -> [_ _ w250]
            frame Default {
            }
            frame 0 {
              n139 = local read "Stage speed (mm/s):"() -> (w240:dbl)
              n140 = Multiply(x=w233, y=w234) -> (x*y=w244:dbl)
              n141 = Divide(x=w244, y=1000.0) -> (x/y=w245:dbl)
              n142 = Divide(x=1.0, y=w245) -> (x/y=w241:dbl)
              n143 = Multiply(x=w240, y=w241) -> (x*y=w239:dbl)
              n144 = To Long Integer(number=w239) -> (32bit integer=w238:i32)
              n145 = Bundle(1, 42, w238, 1) -> (w248:cluster{i32, i32, i32, i32})  [unwired: 1 in]
              n146 = call "Enqueue Message.vi"("Message Data"=w248, "Message"="Update stage speed", "Message Queue"=w247) -> ("error out"=w246:errorcluster)  [unwired: 7 in, 1 out]
            }
            frame 1 {
              n147 = local read "Max position (mm):"() -> (w256:dbl)
              n148 = Divide(x=w250, y=w256) -> (x/y=w257:dbl)
              n149 = Multiply(x="Position (mm):", y=w257) -> (x*y=w258:dbl)
              n150 = To Long Integer(number=w258) -> (32bit integer=w251:i32)
              n151 = Bundle(1, 20, w251, 1) -> (w261:cluster{i32, i32, i32, i32})  [unwired: 1 in]
              n152 = call "Enqueue Message.vi"("Message Data"=w261, "Message"="Go stage", "Message Queue"=w260) -> ("error out"=w259:errorcluster)  [unwired: 7 in, 1 out]
            }
          }
        }
      }
      event "Stop stage", "Stop Test": Value Change {
        n153 = event-data() -> ()  [unwired: 1 in, 1 out]
        n154 = case shown="False" "Stop Test" {
          frame False {
            n155 = local write "Pause Button"(FALSE ("Pause Button")) -> ()
          }
          frame True {
          }
        }
        n156 = Bundle(1, 23, 0, 1) -> (w270:cluster{i32, i32, i32, i32})  [unwired: 1 in]
        n157 = call "Enqueue Message.vi"("Message Data"=w270, "Message"="Stop stage", "Message Queue"=w269) -> ("error out"=w268:errorcluster)  [unwired: 7 in, 1 out]
      }
      event "Contact force (N):": Value Change {
        n158 = event-data() -> ()  [unwired: 1 in, 1 out]
        n159 = local read "Contact force (N):"() -> (w273:fxp<+/-,20,7>)
        n160 = local read "Channel 2 Setpoint"() -> (w278:fxp<+/-,16,5>)
        n161 = local read "Channel 3 Setpoint"() -> (w279:fxp<+/-,16,5>)
        n162 = local read "Channel 1 Setpoint"() -> (w277:fxp<+/-,20,7>)
        n163 = Bundle("Contact force (N):"=w273, "Channel 1 Setpoint"=w277, "Channel 2 Setpoint"=w278, "Channel 3 Setpoint"=w279) -> (w280:T15)  [unwired: 1 in]
        n164 = call "Enqueue Message.vi"("Message Data"=w280, "Message"="Update Setpoints", "Message Queue"=w276) -> ("error out"=w274:errorcluster)  [unwired: 7 in, 1 out]
        n165 = local write "Channel 0 Setpoint"(w273) -> ()
      }
      event "Travel distance (mm):": Value Change {
        # "Keep the inputted travel distance consistent with the range 0-->150 mm"
        n166 = event-data() -> ()  [unwired: 1 in, 1 out]
        n167 = local read "Travel distance (mm):"() -> (w287:dbl)
        n168 = local read "Stage position (mm):"() -> (w288:dbl)
        n169 = Add(x=w288, y=w287) -> (x+y=w281:dbl)
        n170 = Greater?(x=w281, y=0.0) -> (0:w283:bool)
        n171 = Greater Or Equal?(x=150.0, y=w281) -> (x >= y?=w284:bool)
        n172 = And(x=w284, y=w283) -> (x .and. y?=w282:bool)
        n173 = case shown="False" w282 {
          tunnel: w281 -> [w289 w290]
          frame False {
            n174 = local write "Stage stop position (mm):"(w289) -> ()
            n175 = call "Display Message to User"() -> ()  [unwired: 10 in, 2 out]
          }
          frame True {
            n176 = local write "Stage stop position (mm):"(w290) -> ()
          }
        }
      }
      event "Run Test": Value Change {
        n177 = event-data() -> ()  [unwired: 1 in, 1 out]
        n178 = for {
          N: 11 -> [_]
          tunnel: w295 -> [w302]
          tunnel: [w301] -> _
          tunnel: w294 -> [w300]
          tunnel: w293 -> [w299]
          tunnel: w292 -> [w298]
          tunnel: w291 -> [w297]
          i -> [w303]
          n179 = case shown="2" w303 {
            tunnel: w302 -> [_ _ w308 w327 _ _ w343 _ _ _ _ _]
            tunnel: [_ _ w309 w326 _ _ w342 _ _ _ _ _] -> w301
            tunnel: w300 -> [_ _ _ _ _ _ _ _ _ _ _ _]
            tunnel: w299 -> [_ _ w306 _ _ _ _ _ _ _ _ _]
            tunnel: w298 -> [_ _ w307 _ _ _ _ _ _ _ _ _]
            tunnel: w297 -> [_ _ _ _ _ _ w340 _ _ _ _ _]
            frame Default {
            }
            frame 0 {
              w304 = 2
              n180 = property on="Stage speed (mm/s):" class="DigNum (strict)"("DisabledEnum"=w304) -> ()  [unwired: 2 in, 2 out]
              n181 = property on="Position (mm):" class="DigNum (strict)"("DisabledEnum"=w304) -> ()  [unwired: 2 in, 2 out]
              n182 = property on="Contact force (N):" class="DigNum (strict)"("DisabledEnum"=w304) -> ()  [unwired: 2 in, 2 out]
              n183 = property on="Travel distance (mm):" class="DigNum (strict)"("DisabledEnum"=w304) -> ()  [unwired: 2 in, 2 out]
              n184 = property on="Stage speed (mm/s):" class="DigNum (strict)"("DisabledEnum"=w304) -> ()  [unwired: 2 in, 2 out]
              n185 = property on="Start dwell time (s):" class="DigNum (strict)"("DisabledEnum"=w304) -> ()  [unwired: 2 in, 2 out]
              n186 = property on="Stop dwell time (s):" class="DigNum (strict)"("DisabledEnum"=w304) -> ()  [unwired: 2 in, 2 out]
            }
            frame 1 {
              n187 = local read "Stage speed (mm/s):"() -> (w305:dbl)
              n188 = Multiply(x=w307, y=w306) -> (x*y=w313:dbl)
              n189 = Divide(x=w313, y=1000.0) -> (x/y=w312:dbl)
              n190 = Divide(x=1.0, y=w312) -> (x/y=w316:dbl)
              n191 = Multiply(x=w305, y=w316) -> (x*y=w317:dbl)
              n192 = To Long Integer(number=w317) -> (32bit integer=w318:i32)
              n193 = Bundle(1, 42, w318, 1) -> (w311:cluster{i32, i32, i32, i32})  [unwired: 1 in]
              n194 = call "Enqueue Message.vi"("Message Data"=w311, "Message"="Update stage speed", "Message Queue"=w308) -> ("error out"=w309:errorcluster)  [unwired: 7 in, 1 out]
            }
            frame 2 {
              n195 = local read "Channel 3 Setpoint"() -> (w325:fxp<+/-,16,5>)
              n196 = local read "Channel 2 Setpoint"() -> (w324:fxp<+/-,16,5>)
              n197 = local read "Contact force (N):"() -> (w322:fxp<+/-,20,7>)
              n198 = local read "Channel 1 Setpoint"() -> (w323:fxp<+/-,20,7>)
              n199 = Bundle("Contact force (N):"=w322, "Channel 1 Setpoint"=w323, "Channel 2 Setpoint"=w324, "Channel 3 Setpoint"=w325) -> (w328:T15)  [unwired: 1 in]
              n200 = local write "Channel 0 Setpoint"(w322) -> ()
              n201 = call "Enqueue Message.vi"("Message Data"=w328, "Message"="Update Setpoints", "Message Queue"=w327) -> ("error out"=w326:errorcluster)  [unwired: 7 in, 1 out]
            }
            frame 3 {
              n202 = flat-sequence {
                frame #0 {
                  n203 = local write "Number of points"(99999999 ("Number of points")) -> ()
                }
                frame #1 {
                  n204 = local write "Pause Button"(TRUE) -> ()
                  n205 = local write "Clear Button"(TRUE) -> ()
                }
              }
            }
            frame 4 {
              n206 = local read "Start dwell time (s):"() -> (w335:dbl)
              n207 = Multiply(x=w335, y=1000.0) -> (x*y=w334:dbl)
              n208 = Wait (ms)(milliseconds to wait=w334) -> ()  [unwired: 1 out]
            }
            frame 5 {
              n209 = local read "Stage position (mm):"() -> (w336:dbl)
              n210 = local read "Travel distance (mm):"() -> (w338:dbl)
              n211 = local read "Max position (mm):"() -> (w339:dbl)
              n212 = Divide(x=w340, y=w339) -> (x/y=w348:dbl)
              n213 = Add(x=w338, y=w336) -> (x+y=w337:dbl)
              n214 = Multiply(x=w337, y=w348) -> (x*y=w349:dbl)
              n215 = To Long Integer(number=w349) -> (32bit integer=w344:i32)
              n216 = Bundle(1, 20, w344, 1) -> (w341:cluster{i32, i32, i32, i32})  [unwired: 1 in]
              n217 = call "Enqueue Message.vi"("Message Data"=w341, "Message"="Go stage", "Message Queue"=w343) -> ("error out"=w342:errorcluster)  [unwired: 7 in, 1 out]
            }
            frame 6 {
              n218 = while {
                stop <- w368 stop-if-true
                w356 = 100.0 ("y")
                w355 = 100.0 ("x")
                n219 = local read "Stage stop position (mm):"() -> (w360:dbl)
                n220 = shared-variable "NI-cRIO9075-01756F19\\Shared Variables.lvlib\\Stage position"() -> (w357:dbl)  [unwired: 1 in, 1 out]
                n221 = local read "Stop Test"() -> (w364:bool)
                n222 = local read "Test LED"() -> (w366:bool)
                n223 = Multiply(x=w357, y=w355) -> (x*y=w362:dbl)
                n224 = Multiply(x=w360, y=w356) -> (x*y=w361:dbl)
                n225 = Not(x=w366) -> (.not. x?=w363:bool)
                n226 = To Long Integer(number=w362) -> (32bit integer=w359:i32)
                n227 = To Long Integer(number=w361) -> (32bit integer=w354:i32)
                n228 = Divide(x=w354, y=w356) -> (x/y=w353:dbl)
                n229 = Divide(x=w359, y=w355) -> (x/y=w358:dbl)
                n230 = Or(x=w364, y=w363) -> (x .or. y?=w365:bool)
                n231 = To Long Integer(number=w353) -> (32bit integer=w351:i32)
                n232 = To Long Integer(number=w358) -> (32bit integer=w352:i32)
                n233 = Equal?(x=w352, y=w351) -> (x = y?=w367:bool)
                n234 = Or(x=w367, y=w365) -> (x .or. y?=w368:bool)
              }
            }
            frame 7 {
              n235 = local read "Stop Test"() -> (w369:bool)
              n236 = case shown="True" w369 {
                frame False {
                }
                frame True {
                  n237 = local write "Stop dwell time (s):"(0.0 ("Stop dwell time (s):")) -> ()
                }
              }
            }
            frame 8 {
              n238 = local read "Stop dwell time (s):"() -> (w371:dbl)
              n239 = Multiply(x=w371, y=1000.0) -> (x*y=w373:dbl)
              n240 = Wait (ms)(milliseconds to wait=w373) -> ()  [unwired: 1 out]
            }
            frame 9 {
              n241 = local write "Stop Test"(TRUE) -> ()
              n242 = local write "Pause Button"(TRUE) -> ()
            }
            frame 10 {
              w378 = 0
              n243 = local write "Number of points"(500 ("Number of points")) -> ()
              n244 = local write "Travel distance (mm):"(0.0 ("Travel distance (mm):")) -> ()
              n245 = property on="Stage speed (mm/s):" class="DigNum (strict)"("DisabledEnum"=w378) -> ()  [unwired: 2 in, 2 out]
              n246 = property on="Position (mm):" class="DigNum (strict)"("DisabledEnum"=w378) -> ()  [unwired: 2 in, 2 out]
              n247 = property on="Contact force (N):" class="DigNum (strict)"("DisabledEnum"=w378) -> ()  [unwired: 2 in, 2 out]
              n248 = property on="Travel distance (mm):" class="DigNum (strict)"("DisabledEnum"=w378) -> ()  [unwired: 2 in, 2 out]
              n249 = property on="Stage speed (mm/s):" class="DigNum (strict)"("DisabledEnum"=w378) -> ()  [unwired: 2 in, 2 out]
              n250 = property on="Start dwell time (s):" class="DigNum (strict)"("DisabledEnum"=w378) -> ()  [unwired: 2 in, 2 out]
              n251 = property on="Stop dwell time (s):" class="DigNum (strict)"("DisabledEnum"=w378) -> ()  [unwired: 2 in, 2 out]
            }
          }
        }
      }
      event User Event {
        # "The Message Handling Loop processed an \"Exit\" message, which fired this event to stop the Event Handling Loop."
        n252 = event-data() -> ()  [unwired: 1 in, 1 out]
      }
      event "Save As Button", "Save Results": Value Change {
        # "When Save As is pressed, V*, Force, and Position are saved."
        n253 = event-data() -> ()  [unwired: 1 in, 1 out]
        n254 = stacked-sequence {
          frame #0 {
            n255 = call "File Dialog"() -> ("selected path"=w382:path)  [unwired: 12 in, 3 out]
            n256 = local read "Stage position (mm)"() -> (w391:cluster{dbl[], dbl[]})
            n257 = local read "Roller position (mm)"() -> (w390:cluster{dbl[], dbl[]})
            n258 = local read "Force (N)"() -> (w388:cluster{dbl[], dbl[]})
            n259 = local read "V*"() -> (w389:cluster{dbl[], dbl[]})
            n260 = Unbundle(w391) -> (w407:dbl[], w408:dbl[])
            n261 = Unbundle(w388) -> (w393:dbl[])  [unwired: 1 out]
            n262 = Unbundle(w390) -> (w392:dbl[])  [unwired: 1 out]
            n263 = Unbundle(w389) -> (w395:dbl[])  [unwired: 1 out]
            n264 = Array Max & Min(array=w407) -> (min value=w405:dbl)  [unwired: 3 out]
            n265 = Subtract(x=w407, y=w405) -> (x-y=w406:dbl[])
            n266 = Build Array(w406, w408, w393, w392, w395) -> (w411:dbl[][])
            n267 = Build Array("Time (s)" ("element"), "Stage position (mm)" ("element"), "Force (N)" ("element"), "Roller position (mm)" ("element"), "V* (V)" ("element")) -> (w397:string[])
            n268 = Strip Path(path=w382) -> (stripped path=w383:path, name=w386:string)
            n269 = Transpose 2D Array(2D array=w411) -> (transposed array=w409:dbl[][])
            n270 = Concatenate Strings(w386, ".txt" ("name or relative path")) -> (w384:string)
            n271 = Array To Spreadsheet String(array=w397, 3:"%s") -> (spreadsheet string=w400:string)  [unwired: 1 in]
            n272 = local write "Pause Button"(TRUE) -> ()
            n273 = local write "Stop Test"(TRUE) -> ()
            n274 = Build Path(base path=w383, name or relative path=w384) -> (appended path=w380:path)
            "path" <- w380
            n275 = Open/Create/Replace File(file path (use dialog)=w380, operation (0:open)=T7."replace or create with confirmation") -> (refnum out=w381:refnum<file>, error out=w415:errorcluster)  [unwired: 4 in, 1 out]
            n276 = Array To Spreadsheet String(array=w409, 3:"%g" ("format string")) -> (spreadsheet string=w399:string)  [unwired: 1 in]
            n277 = Concatenate Strings(w400, w399) -> (w398:string)
            n278 = Write to Text File(file (use dialog)=w381, text=w398, error in=w415) -> (refnum out=w413:refnum<file>, error out=w414:errorcluster)  [unwired: 2 out]
            n279 = Close File(refnum=w413, error in=w414) -> ()  [unwired: 2 out]
          }
          frame #1 {
            n280 = local read "Save Results"() -> (w417:bool)
            n281 = case shown="True" w417 {
              frame False {
              }
              frame True {
                n282 = Get Date/Time In Seconds() -> (seconds since 1Jan1904=w428:timestamp)
                n283 = local read "Contact force (N):"() -> (w425:fxp<+/-,20,7>)
                n284 = local read "Travel distance (mm):"() -> (w423:dbl)
                n285 = local read "Stage speed (mm/s):"() -> (w422:dbl)
                n286 = local read "path"() -> (w434:path)
                n287 = local read "Start dwell time (s):"() -> (w421:dbl)
                n288 = local read "Stop dwell time (s):"() -> (w420:dbl)
                n289 = Get Date/Time String(seconds (now)=w428) -> (date string=w427:string, time string=w426:string)  [unwired: 2 in]
                n290 = Build Array(w427, w426) -> (w429:string[])
                n291 = Strip Path(path=w434) -> (stripped path=w440:path, name=w439:string)
                n292 = To Double Precision Float(number=w425) -> (double precision float=w424:dbl)
                n293 = Array To Spreadsheet String(array=w429, 3:"%s") -> (spreadsheet string=w430:string)  [unwired: 1 in]
                n294 = Build Array("Setpoint force (N)" ("element"), "Travel distance (mm)" ("element"), "Stage speed (mm/s)" ("element"), "Start dwell time (s)" ("element"), "Stop dwell time (s)" ("element")) -> (w443:string[])
                n295 = Build Array(w424, w423, w422, w421, w420) -> (w419:dbl[])
                n296 = Build Array(w419) -> (w418:dbl[][])
                n297 = Search and Replace String(input string=w439, search string=".txt" ("name or relative path"), replace string="_params.txt" ("name or relative path")) -> (result string=w437:string)  [unwired: 5 in, 3 out]
                n298 = Array To Spreadsheet String(array=w443, 3:"%s") -> (spreadsheet string=w450:string)  [unwired: 1 in]
                n299 = Array To Spreadsheet String(array=w418, 3:"%g" ("format string")) -> (spreadsheet string=w451:string)  [unwired: 1 in]
                n300 = Build Path(base path=w440, name or relative path=w437) -> (appended path=w435:path)
                n301 = Open/Create/Replace File(file path (use dialog)=w435, operation (0:open)=T7."replace or create with confirmation") -> (refnum out=w453:refnum<file>, error out=w442:errorcluster)  [unwired: 4 in, 1 out]
                n302 = Concatenate Strings(w450, w451) -> (w432:string)
                n303 = Concatenate Strings(w430, w432) -> (w431:string)
                n304 = Write to Text File(file (use dialog)=w453, text=w431, error in=w442) -> (refnum out=w455:refnum<file>, error out=w441:errorcluster)  [unwired: 2 out]
                n305 = Close File(refnum=w455, error in=w441) -> ()  [unwired: 2 out]
              }
            }
          }
          frame #2 {
            n306 = local write "Save As Button"(FALSE ("Pause Button")) -> ()
            n307 = local write "Save Results"(FALSE ("Save Results")) -> ()
          }
        }
      }
      event "Clear Button": Value Change {
        # "When the Clear button is pressed, all data are erased."
        n308 = event-data() -> ()  [unwired: 1 in, 1 out]
        n309 = local write "Pause Button"(TRUE) -> ()
      }
    }
    n310 = case shown="Error" w33 {
      tunnel: [w36 TRUE ("Discard?")] -> w34
      tunnel: w35 -> [w36 _]
      tunnel: w31 -> [_ w37]
      frame No Error {
      }
      frame Error {
        # "On error, send Exit message, and stop loop."
        n311 = call "Enqueue Message.vi"("Priority Message? (F)"=TRUE ("Discard?"), "Message"="Exit", "Message Queue"=w37) -> ()  [unwired: 7 in, 2 out]
      }
    }
  }
  n312 = while {
    tunnel: w11 -> [w464]
    tunnel: w19 -> [w469]
    shift-right: [w459] -> w23
    shift-left: w16 -> [w468]
    shift-right: [w462] -> _
    shift-left: T5 {"Switch to Safe State Ref"=refnum, "Run Manual Ref"=refnum, "Stop Manual Ref"=refnum, "Run Control Ref"=refnum, "Stop Control Ref"=refnum, "Update Control Configurations Ref"=refnum, "Ch 0 Setpoint Ref"=refnum, "Ch 1 Setpoint Ref"=refnum, "Ch 2 Setpoint Ref"=refnum, "Ch 3 Setpoint Ref"=refnum, "Ch 0 Manual Ref"=refnum, "Ch 1 Manual Ref"=refnum, "Ch 2 Manual Ref"=refnum, "Ch 3 Manual Ref"=refnum, "Control Configurations Ref"=refnum, "Control period (ticks) Ref"=refnum, "Roller control"=refnum, "Disable roller control"=refnum, "Test control"=refnum, "Disable test control"=refnum, "Motion Observer"=refnum, "Digital Controller"=refnum} ("Measurement UI Controls") -> [w463]
    stop <- w470 stop-if-true
    # "UI Message Loop"
    n313 = call "Dequeue Message.vi"("error in (no error)"=w468, "Message Queue"=w464) -> ("error out"=w467:errorcluster, "Message Data"=w465:variant, "Message"=w466:string, "dup Message Queue"=w461:refnum<queue>)  [unwired: 6 in]
    n314 = case "Message Cases" shown="\"Update Custom Controller\"" w466 {
      selector: w466 -> [_ _ _ _ _ _ _ _ _ w616 _ _ _ _ w684 _ w750 _ _ _ _ _ _ _ _ _ w883]
      tunnel: w461 -> [w472 w486 _ _ w556 _ w574 _ w592 w617 _ _ _ _ _ _ w754 _ _ _ _ _ _ _ w868 _ _]
      tunnel: w467 -> [w474 w504 w531 w540 w561 w572 w576 w581 w612 w619 w637 w648 w659 w672 w685 w709 w764 w785 w795 w807 w817 w831 w843 w854 w873 w878 _]
      tunnel: [w473 w487 w531 w540 w555 w572 w575 w580 w595 w618 w636 w647 w658 w671 w686 w708 w765 w783 w793 w806 w816 w830 w842 w855 w874 w877 w881] -> w460
      tunnel: [_ _ _ _ _ _ _ _ _ _ _ _ _ _ _ _ _ _ _ _ _ _ _ _ TRUE _ _] -> w470
      tunnel: w465 -> [_ _ _ _ _ _ _ _ w610 _ _ _ _ w673 w683 w707 w762 w782 w794 w805 w818 w828 w840 w853 _ _ _]
      tunnel: w469 -> [_ _ _ _ _ _ _ _ _ _ _ _ _ _ _ _ _ _ _ _ _ _ _ _ w872 _ _]
      tunnel: w463 -> [w475 w503 w530 w551 w560 w571 w578 w582 w607 w620 w638 w649 w660 w674 w687 w706 w766 w784 w796 w808 w820 w832 w844 w856 w870 w876 w879]
      tunnel: [w475 w502 w530 w551 w560 w571 w578 w582 w607 w620 w638 w649 w660 w674 w687 w706 w766 w784 w796 w808 w820 w832 w844 w856 w870 w876 w879] -> w462
      frame "Initialize" {
        # "Initialize - Send 'Initialize UI Refs' message to get the UI references bundled and initialized appropriately."
        n315 = call "Enqueue Message.vi"("error in (no error)"=w474, "Message"="Initialize UI Refs", "Message Queue"=w472) -> ("error out"=w473:errorcluster)  [unwired: 7 in, 1 out]
      }
      frame "Initialize UI Refs" {
        # "Send a message to disable them all, since there is no connection at the start."
        # "Initialize UI Refs - Bundle up a cluster of references of all UI elements that are programmatically manipulated."
        n316 = control-ref of="Switch to Safe State"() -> (w501:refnum<vi>)
        n317 = control-ref of="Run Manual"() -> (w500:refnum<vi>)
        n318 = control-ref of="Stop Manual"() -> (w499:refnum<vi>)
        n319 = control-ref of="Run Control"() -> (w498:refnum<vi>)
        n320 = control-ref of="Stop Control"() -> (w497:refnum<vi>)
        n321 = control-ref of="Update Control Configuration"() -> (w496:refnum<vi>)
        n322 = control-ref of="Roller control"() -> (w482:refnum<vi>)
        n323 = control-ref of="Disable roller control"() -> (w481:refnum<vi>)
        n324 = control-ref of="Test control"() -> (w480:refnum<vi>)
        n325 = control-ref of="Disable test control"() -> (w479:refnum<vi>)
        n326 = control-ref of="Motion Observer"() -> (w478:refnum<vi>)
        n327 = control-ref of="Motion Observer"() -> (w476:refnum<vi>)
        n328 = control-ref of="Control period (ticks)"() -> (w483:refnum<vi>)
        n329 = control-ref of="Digital Controller"() -> (w477:refnum<vi>)
        n330 = control-ref of="Channel 0 Setpoint"() -> (w495:refnum<vi>)
        n331 = control-ref of="Channel 1 Setpoint"() -> (w494:refnum<vi>)
        n332 = control-ref of="Channel 2 Setpoint"() -> (w493:refnum<vi>)
        n333 = control-ref of="Channel 3 Setpoint"() -> (w492:refnum<vi>)
        n334 = control-ref of="Channel 0 Manual Value"() -> (w491:refnum<vi>)
        n335 = control-ref of="Channel 1 Manual Value"() -> (w490:refnum<vi>)
        n336 = control-ref of="Channel 2 Manual Value"() -> (w489:refnum<vi>)
        n337 = control-ref of="Channel 3 Manual Value"() -> (w488:refnum<vi>)
        n338 = control-ref of="Control Configurations"() -> (w484:refnum<vi>)
        n339 = call "Enqueue Message.vi"("error in (no error)"=w504, "Message"="Disable Controls", "Message Queue"=w486) -> ("error out"=w487:errorcluster)  [unwired: 7 in, 1 out]
        n340 = Bundle By Name(cluster=w503, "Switch to Safe State Ref"=w501, "Run Manual Ref"=w500, "Stop Manual Ref"=w499, "Run Control Ref"=w498, "Stop Control Ref"=w497, "Update Control Configurations Ref"=w496, "Ch 0 Setpoint Ref"=w495, "Ch 1 Setpoint Ref"=w494, "Ch 2 Setpoint Ref"=w493, "Ch 3 Setpoint Ref"=w492, "Ch 0 Manual Ref"=w491, "Ch 1 Manual Ref"=w490, "Ch 2 Manual Ref"=w489, "Ch 3 Manual Ref"=w488, "Control Configurations Ref"=w484, "Digital Controller"=w477, "Motion Observer"=w476, "Control period (ticks) Ref"=w483, "Roller control"=w482, "Disable roller control"=w481, "Test control"=w480, "Disable test control"=w479, "Motion Observer"=w478) -> (w502:T5)
      }
      frame "Disable Controls" {
        w512 = 0
        # "With the control options disabled, the only thing the user can do is Connect. Make sure the IP address string and connect button are enabled."
        # "Disable All Controls - Set all controls in the UI Refs cluster to \"Disabled and Grayed Out\"."
        n341 = Unbundle(w530) -> ("Switch to Safe State Ref"=w529:refnum<vi>, "Run Manual Ref"=w528:refnum<vi>, "Stop Manual Ref"=w527:refnum<vi>, "Run Control Ref"=w526:refnum<vi>, "Stop Control Ref"=w525:refnum<vi>, "Update Control Configurations Ref"=w524:refnum<vi>, "Ch 0 Setpoint Ref"=w523:refnum<vi>, "Ch 1 Setpoint Ref"=w522:refnum<vi>, "Ch 2 Setpoint Ref"=w521:refnum<vi>, "Ch 3 Setpoint Ref"=w520:refnum<vi>, "Ch 0 Manual Ref"=w519:refnum<vi>, "Ch 1 Manual Ref"=w518:refnum<vi>, "Ch 2 Manual Ref"=w517:refnum<vi>, "Ch 3 Manual Ref"=w516:refnum<vi>, "Control Configurations Ref"=w515:refnum<vi>, "Control period (ticks) Ref"=w511:refnum<vi>, "Roller control"=w510:refnum<vi>, "Disable roller control"=w509:refnum<vi>, "Test control"=w508:refnum<vi>, "Disable test control"=w507:refnum<vi>, "Motion Observer"=w506:refnum<vi>, "Digital Controller"=w505:refnum<vi>)
        n342 = Build Array(w529, w528, w527, w526, w525, w524, w523, w522, w521, w520, w519, w518, w517, w516, w515, w511, w510, w509, w508, w507, w506, w505) -> (w514:refnum<vi>[])
        n343 = call "Set Enable State on Multiple Controls.vi"("Enable?"=FALSE, "Controls"=w514) -> ()  [unwired: 10 in]
        n344 = property on="Controller Address" class="Str"("DisabledEnum"=w512) -> ()  [unwired: 2 in, 2 out]
        n345 = property on="Connect to Controller" class="Bool"("DisabledEnum"=w512) -> ()  [unwired: 2 in, 2 out]
      }
      frame "Enable Configuration Controls" {
        w552 = 2
        # "Once connected, the user shouldn't be able to change the connection settings unless he gets disconnected."
        # "Enable Configuration Controls - After successful connection, ensure appropriate controls are enabled."
        n346 = Unbundle By Name(w551) -> ("Update Control Configurations Ref"=w550:refnum<vi>, "Ch 0 Setpoint Ref"=w549:refnum<vi>, "Ch 1 Setpoint Ref"=w548:refnum<vi>, "Ch 2 Setpoint Ref"=w547:refnum<vi>, "Ch 3 Setpoint Ref"=w546:refnum<vi>, "Ch 0 Manual Ref"=w545:refnum<vi>, "Ch 1 Manual Ref"=w544:refnum<vi>, "Ch 2 Manual Ref"=w543:refnum<vi>, "Ch 3 Manual Ref"=w542:refnum<vi>, "Control Configurations Ref"=w541:refnum<vi>, "Digital Controller"=w539:refnum<vi>, "Motion Observer"=w538:refnum<vi>, "Control period (ticks) Ref"=w537:refnum<vi>, "Roller control"=w536:refnum<vi>, "Disable roller control"=w535:refnum<vi>, "Test control"=w534:refnum<vi>, "Disable test control"=w533:refnum<vi>, "Motion Observer"=w532:refnum<vi>)
        n347 = Build Array(w550, w549, w548, w547, w546, w545, w544, w543, w542, w541, w539, w538, w537, w536, w535, w534, w533, w532) -> (w554:refnum<vi>[])
        n348 = call "Set Enable State on Multiple Controls.vi"("Enable?"=TRUE, "Controls"=w554) -> ()  [unwired: 10 in]
        n349 = property on="Controller Address" class="Str"("DisabledEnum"=w552) -> ()  [unwired: 2 in, 2 out]
        n350 = property on="Connect to Controller" class="Bool"("DisabledEnum"=w552) -> ()  [unwired: 2 in, 2 out]
      }
      frame "Connect" {
        # "Connect - Attempt to connect to both streams, and the variables, on the RT target."
        n351 = call "UI - Initiate Connection.vi"("error in (no error)"=w561, "Controller Address"="Controller Address", "Message Queue"=w556) -> ("error out"=w558:errorcluster, "Connected?"=w557:bool)  [unwired: 7 in]
        "Connected?" <- w557
        n352 = case shown="True" w557 {
          tunnel: w558 -> [w562 w566]
          tunnel: w556 -> [_ w565]
          tunnel: [w562 w564] -> w555
          frame False {
          }
          frame True {
            n353 = call "Enqueue Message.vi"("error in (no error)"=w566, "Message"="Enable Configuration Controls", "Message Queue"=w565) -> ("error out"=w564:errorcluster)  [unwired: 7 in, 1 out]
          }
        }
      }
      frame "Close Connections" {
        # "Close Connections - Close the connections shared with the Monitoring Loop."
        n354 = global read "Global - UI Stream and Variable Connections.vi" "UI Command Stream"() -> (w570:refnum<k21>)
        n355 = global read "Global - UI Stream and Variable Connections.vi" "RT Message Stream"() -> (w569:refnum<k21>)
        n356 = global read "Global - UI Stream and Variable Connections.vi" "Variable References"() -> (w568:T10)
        n357 = local write "Connected?"(FALSE ("Connected?")) -> ()
        n358 = Destroy Stream Endpoint(11:w570) -> ()  [unwired: 1 in, 1 out]
        n359 = Destroy Stream Endpoint(11:w569) -> ()  [unwired: 1 in, 1 out]
        n360 = call "Close Variable Connections.vi"("Variable References"=w568) -> ()  [unwired: 11 in]
      }
      frame "Disconnect UI" {
        # "Disconnect UI - Something has gone wrong with the connection. Reinitialize the UI to its disconnected state."
        n361 = local write "Connected?"(FALSE ("Connected?")) -> ()
        n362 = call "Enqueue Message.vi"("error in (no error)"=w576, "Message"="Disable Controls", "Message Queue"=w574) -> ("error out"=w575:errorcluster)  [unwired: 7 in, 1 out]
      }
      frame "Get Settings from FPGA" {
        # "Get Settings from FPGA - Send a command to the RT to retrieve all current FPGA Main VI parameter values and send them back to the UI."
        n363 = local read "Connected?"() -> (w579:bool)
        n364 = case shown="True" w579 {
          tunnel: w581 -> [w583 w587]
          tunnel: [w583 w586] -> w580
          frame False {
            # "Don't bother trying to send a message to the RT system if UI Main VI isn't even connected"
          }
          frame True {
            n365 = global read "Global - UI Stream and Variable Connections.vi" "UI Command Stream"() -> (w584:refnum<k21>)
            n366 = shared-variable-write(w584, w587, T16 {"Message"="Send FPGA Configuration to UI", "Message Data"=variant} ("data in")) -> (w586:errorcluster)  [unwired: 1 in, 2 out]
          }
        }
      }
      frame "Initial UI Values" {
        # "Initial UI Values - These are the current values of the FPGA Main VI's R/W controls. They are used to initialize the panel of UI Main VI upon successful connection to the RT target."
        # "Set values of all manual and setpoint controls via reference."
        n367 = Variant To Data(error in=w612, type=T17 {"FPGA State"=enum."Safe State", "Manual Values"={"Channel 0"=0.0, "Channel 1"=0.0, "Channel 2"=0.0, "Channel 3"=0.0}, "Setpoints"={"Channel 0"=0.0, "Channel 1"=0.0, "Channel 2"=0.0, "Channel 3"=0.0}, "Control Configurations"=[]} ("All FPGA Configuration Values"), Variant=w610) -> (data=w608:T17, error out=w611:errorcluster)
        n368 = Unbundle By Name(w607) -> ("Ch 0 Setpoint Ref"=w606:refnum<vi>, "Ch 1 Setpoint Ref"=w605:refnum<vi>, "Ch 2 Setpoint Ref"=w604:refnum<vi>, "Ch 3 Setpoint Ref"=w603:refnum<vi>, "Ch 0 Manual Ref"=w602:refnum<vi>, "Ch 1 Manual Ref"=w601:refnum<vi>, "Ch 2 Manual Ref"=w600:refnum<vi>, "Ch 3 Manual Ref"=w599:refnum<vi>)
        n369 = Unbundle By Name(w608) -> ("Setpoints"=w590:T11, "Manual Values"=w588:T11, "Control Configurations"=w596:T3[], "FPGA State"=w593:T18)
        n370 = Build Array(w606, w605, w604, w603, w602, w601, w600, w599) -> (w598:refnum<vi>[])
        n371 = To Variant(anything=w588) -> (Variant=w589:variant)
        n372 = To Variant(anything=w590) -> (Variant=w591:variant)
        n373 = local write "Current FPGA Control Mode"(w593) -> ()
        n374 = Build Array(w591, w589) -> (w597:variant[])
        n375 = local write "Control Configurations"(w596) -> ()
        n376 = for {
          tunnel: w598 -> [w614] mode=indexing
          tunnel: w597 -> [w613] mode=indexing
          n377 = property class="DigNum"(reference=w614, "Value"=w613) -> ()  [unwired: 1 in, 2 out]
        }
        n378 = call "Enqueue Message.vi"("error in (no error)"=w611, "Message Data"=w593, "Message"="Update Display Mode", "Message Queue"=w592) -> ("error out"=w595:errorcluster)  [unwired: 6 in, 1 out]
      }
      frame "Run Control", "Run Manual", "Run Safe State", "Stop Control", "Stop Manual" {
        # "Run/Stop buttons - Send a command to switch the FPGA into the appropriate state. Send a message to update this UI to reflect the new state."
        n379 = local read "Connected?"() -> (w615:bool)
        n380 = case shown="True" w615 {
          tunnel: w619 -> [w621 w631]
          tunnel: [w621 w627] -> w618
          tunnel: w617 -> [_ w626]
          tunnel: w616 -> [_ w625]
          frame False {
            # "Don't bother trying to send a message to the RT system if UI Main VI isn't even connected"
          }
          frame True {
            # "Run Manual and Run Control switch into their respective states. Anything else switches to Safe State."
            n381 = case shown="\"Run Control\"" w625 {
              tunnel: [FPGA_State."Safe State" ("FPGA State") FPGA_State."Control (PID)" ("FPGA State") FPGA_State."Manual" ("FPGA State")] -> w622
              frame "Safe State", "Stop Control", "Stop Manual", Default {
              }
              frame "Run Control" {
              }
              frame "Run Manual" {
              }
            }
            n382 = global read "Global - UI Stream and Variable Connections.vi" "UI Command Stream"() -> (w623:refnum<k21>)
            n383 = Bundle("Update FPGA State", "FPGA State"=w622) -> (w628:cluster{string, "FPGA State":T18})  [unwired: 1 in]
            n384 = shared-variable-write(w623, w631, w628) -> (w630:errorcluster)  [unwired: 1 in, 2 out]
            n385 = call "Enqueue Message.vi"("error in (no error)"=w630, "Message Data"=w622, "Message"="Update Display Mode", "Message Queue"=w626) -> ("error out"=w627:errorcluster)  [unwired: 6 in, 1 out]
          }
        }
      }
      frame "Update Control period" {
        n386 = local read "Connected?"() -> (w635:bool)
        n387 = case shown="True" w635 {
          tunnel: w637 -> [w639 w645]
          tunnel: [w639 w644] -> w636
          frame False {
            # "Don't bother trying to send a message to the RT system if UI Main VI isn't even connected"
          }
          frame True {
            n388 = global read "Global - UI Stream and Variable Connections.vi" "UI Command Stream"() -> (w641:refnum<k21>)
            n389 = local read "Control period (ticks)"() -> (w640:u32)
            n390 = Bundle("Update Control period", "Control period (ticks)"=w640) -> (w642:cluster{string, "Control period (ticks)":u32})  [unwired: 1 in]
            n391 = shared-variable-write(w641, w645, w642) -> (w644:errorcluster)  [unwired: 1 in, 2 out]
          }
        }
      }
      frame "Update Control Configuration" {
        # "Update Control Configuration - Send all control configurations to RT to be sent down to the FPGA."
        n392 = local read "Connected?"() -> (w646:bool)
        n393 = case shown="True" w646 {
          tunnel: w648 -> [w650 w656]
          tunnel: [w650 w655] -> w647
          frame False {
            # "Don't bother trying to send a message to the RT system if UI Main VI isn't even connected"
          }
          frame True {
            n394 = global read "Global - UI Stream and Variable Connections.vi" "UI Command Stream"() -> (w651:refnum<k21>)
            n395 = Bundle("Update Control Configurations", "Control Configurations"="Control Configurations") -> (w653:cluster{string, "Control Configurations":T3[]})  [unwired: 1 in]
            n396 = shared-variable-write(w651, w656, w653) -> (w655:errorcluster)  [unwired: 1 in, 2 out]
          }
        }
      }
      frame "Update Custom Controller" {
        # "Update Control Configuration - Send all control configurations to RT to be sent down to the FPGA."
        n397 = local read "Connected?"() -> (w657:bool)
        n398 = case shown="True" w657 {
          tunnel: w659 -> [w661 w669]
          tunnel: [w661 w668] -> w658
          frame False {
            # "Don't bother trying to send a message to the RT system if UI Main VI isn't even connected"
          }
          frame True {
            n399 = global read "Global - UI Stream and Variable Connections.vi" "UI Command Stream"() -> (w665:refnum<k21>)
            n400 = Bundle("Digital Controller"="Digital Controller", "Motion Observer"="Motion Observer") -> (w662:T19)  [unwired: 1 in]
            n401 = Bundle("Update Custom Controller", w662) -> (w666:T20)  [unwired: 1 in]
            n402 = shared-variable-write(w665, w669, w666) -> (w668:errorcluster)  [unwired: 1 in, 2 out]
          }
        }
      }
      frame "Update stage speed" {
        n403 = local read "Connected?"() -> (w670:bool)
        n404 = case shown="True" w670 {
          tunnel: w672 -> [w675 w681]
          tunnel: [w675 w680] -> w671
          tunnel: w673 -> [_ w676]
          frame False {
            # "Don't bother trying to send a message to the RT system if UI Main VI isn't even connected"
          }
          frame True {
            n405 = global read "Global - UI Stream and Variable Connections.vi" "UI Command Stream"() -> (w677:refnum<k21>)
            n406 = Bundle("Update stage speed", "Message Data"=w676) -> (w678:cluster{string, "Message Data":variant})  [unwired: 1 in]
            n407 = shared-variable-write(w677, w681, w678) -> (w680:errorcluster)  [unwired: 1 in, 2 out]
          }
        }
      }
      frame "Update Manual Values", "Update Setpoints" {
        # "Update Manual Values/Setpoints - Send all manual values/setpoints to RT to be sent down to the FPGA."
        n408 = local read "Connected?"() -> (w682:bool)
        n409 = case shown="True" w682 {
          tunnel: [w688 w694] -> w686
          tunnel: w685 -> [w688 w692]
          tunnel: w684 -> [_ w691]
          tunnel: w683 -> [_ w690]
          frame False {
            # "Don't bother trying to send a message to the RT system if UI Main VI isn't even connected"
          }
          frame True {
            n410 = global read "Global - UI Stream and Variable Connections.vi" "UI Command Stream"() -> (w689:refnum<k21>)
            n411 = Bundle(w691, "Message Data"=w690) -> (w693:cluster{string, "Message Data":variant})  [unwired: 1 in]
            n412 = shared-variable-write(w689, w692, w693) -> (w694:errorcluster)  [unwired: 1 in, 2 out]
          }
        }
      }
      frame "Update Display Mode" {
        # "Update Display Mode - Enable/Disable Controls appropriately for the new display mode."
        n413 = Variant To Data(error in=w709, type=FPGA_State."Safe State" ("FPGA State"), Variant=w707) -> (data=w705:T18, error out=w708:errorcluster)
        n414 = Unbundle By Name(w706) -> ("Switch to Safe State Ref"=w704:refnum<vi>, "Run Manual Ref"=w703:refnum<vi>, "Stop Manual Ref"=w702:refnum<vi>, "Run Control Ref"=w701:refnum<vi>, "Stop Control Ref"=w700:refnum<vi>, "Roller control"=w698:refnum<vi>, "Disable roller control"=w697:refnum<vi>, "Test control"=w696:refnum<vi>, "Disable test control"=w695:refnum<vi>)
        n415 = case shown="\"Safe State\"" w705 {
          tunnel: w704 -> [w718 w731 w742]
          tunnel: w703 -> [w714 w730 w744]
          tunnel: w702 -> [w717 w729 w741]
          tunnel: w701 -> [w716 w727 w743]
          tunnel: w700 -> [w715 w728 w740]
          tunnel: w698 -> [w712 w726 w739]
          tunnel: w697 -> [w711 w725 w738]
          tunnel: w696 -> [w713 w724 w737]
          tunnel: w695 -> [w710 w723 w736]
          frame "Control (PID)" {
            n416 = Build Array "Controls to Enable"(w718, w715, w714, w712, w710) -> (w722:refnum<vi>[])
            n417 = Build Array "Controls to Disable"(w717, w716, w713, w711) -> (w720:refnum<vi>[])
            n418 = call "Set Enable State on Multiple Controls.vi"("Enable?"=FALSE, "Controls"=w720) -> ()  [unwired: 10 in]
            n419 = call "Set Enable State on Multiple Controls.vi"("Enable?"=TRUE, "Controls"=w722) -> ()  [unwired: 10 in]
          }
          frame "Manual" {
            n420 = Build Array "Controls to Enable"(w731, w729, w727, w725, w724) -> (w735:refnum<vi>[])
            n421 = Build Array "Controls to Disable"(w730, w728, w726, w723) -> (w733:refnum<vi>[])
            n422 = call "Set Enable State on Multiple Controls.vi"("Enable?"=FALSE, "Controls"=w733) -> ()  [unwired: 10 in]
            n423 = call "Set Enable State on Multiple Controls.vi"("Enable?"=TRUE, "Controls"=w735) -> ()  [unwired: 10 in]
          }
          frame "Safe State" {
            # "This frame runs when FPGA is in Safe State. Only enable the two run buttons."
            n424 = Build Array "Controls to Enable"(w744, w743, w739, w737) -> (w748:refnum<vi>[])
            n425 = Build Array "Controls to Disable"(w742, w741, w740, w738, w736) -> (w746:refnum<vi>[])
            n426 = call "Set Enable State on Multiple Controls.vi"("Enable?"=FALSE, "Controls"=w746) -> ()  [unwired: 10 in]
            n427 = call "Set Enable State on Multiple Controls.vi"("Enable?"=TRUE, "Controls"=w748) -> ()  [unwired: 10 in]
          }
        }
      }
      frame "Critical Error", "Log-Only Error", "Non-Critical Error", "RT Error" {
        # "Error - Display message in status indicator on panel.  If it's a critical error, shut down this VI with an 'Exit' message."
        n428 = case shown="Default" w750 {
          selector: w750 -> [_ w768]
          tunnel: ["UI Error" w768] -> w749
          frame Default {
          }
          frame "RT Error" {
          }
        }
        n429 = Variant To Data(error in=w764, type=errorcluster {"status"=FALSE, "code"=0, "source"=""} ("error constant"), Variant=w762) -> (data=w757:errorcluster, error out=w763:errorcluster)
        n430 = Unbundle By Name(w757) -> ("code"=w756:i32, "source"=w760:string)
        n431 = Format Date/Time String() -> (date/time string=w759:string)  [unwired: 3 in]
        n432 = Format Into String(format string="\n%s: %s %d - %s", w759, w749, w756, w760) -> (resulting string=w751:string)  [unwired: 2 in, 1 out]
        n433 = call "Enqueue Message.vi"("error in (no error)"=w763, "Message Data"=w751, "Message"="Update System Status", "Message Queue"=w754) -> ("error out"=w755:errorcluster, "dup Message Queue"=w753:refnum<queue>)  [unwired: 6 in]
        n434 = case shown="Default" w750 {
          tunnel: w755 -> [w769 w773]
          tunnel: w753 -> [_ w771]
          tunnel: [w769 w772] -> w765
          frame Default {
          }
          frame "Critical Error" {
            n435 = call "Enqueue Message.vi"("error in (no error)"=w773, "Message"="Exit", "Message Queue"=w771) -> ("error out"=w772:errorcluster)  [unwired: 7 in, 1 out]
          }
        }
      }
      frame "Update System Status" {
        # "Code Recommended - The code below ensures that the System Status string value does not become too large.  It uses the same maximum size as the RT error log to determine whether or not to remove the last half of the log string. Change this logic if you wish to maintain more/less of the information in the System Status string."
        # "Update System Status - Add a new string to the beginning of the System Status string on the UI."
        n436 = Variant To Data(error in=w785, type="", Variant=w782) -> (data=w779:string, error out=w783:errorcluster)
        n437 = local read "System Status"() -> (w777:string)
        n438 = global read "Global - Configuration Options.vi" "Error Log Max Size (bytes)"() -> (w775:i64)
        n439 = String Length(string=w777) -> (length=w778:i32)
        n440 = Greater?(x=w778, y=w775) -> (0:w776:bool)
        n441 = case shown="True" w776 {
          tunnel: w777 -> [w786 w790]
          tunnel: w775 -> [_ w789]
          tunnel: [w786 w791] -> w774
          frame False {
          }
          frame True {
            n442 = Divide(x=w789, y=i64 2) -> (x/y=w788:dbl)
            n443 = String Subset(string=w790, length (rest)=w788) -> (substring=w791:string)  [unwired: 1 in]
          }
        }
        n444 = Concatenate Strings(w779, w774) -> (→"System Status":string)
      }
      frame "Home roller" {
        n445 = local read "Connected?"() -> (w792:bool)
        n446 = case shown="True" w792 {
          tunnel: [w797 w803] -> w793
          tunnel: w795 -> [w797 w801]
          tunnel: w794 -> [_ w800]
          frame False {
            # "Don't bother trying to send a message to the RT system if UI Main VI isn't even connected"
          }
          frame True {
            n447 = global read "Global - UI Stream and Variable Connections.vi" "UI Command Stream"() -> (w799:refnum<k21>)
            n448 = Bundle("Message"="Update Manual Values", "Message Data"=w800) -> (w802:T16)  [unwired: 1 in]
            n449 = shared-variable-write(w799, w801, w802) -> (w803:errorcluster)  [unwired: 1 in, 2 out]
          }
        }
      }
      frame "Contact roller" {
        n450 = local read "Connected?"() -> (w804:bool)
        n451 = case shown="True" w804 {
          tunnel: [w809 w815] -> w806
          tunnel: w807 -> [w809 w813]
          tunnel: w805 -> [_ w812]
          frame False {
            # "Don't bother trying to send a message to the RT system if UI Main VI isn't even connected"
          }
          frame True {
            n452 = global read "Global - UI Stream and Variable Connections.vi" "UI Command Stream"() -> (w811:refnum<k21>)
            n453 = Bundle("Message"="Update Manual Values", "Message Data"=w812) -> (w814:T16)  [unwired: 1 in]
            n454 = shared-variable-write(w811, w813, w814) -> (w815:errorcluster)  [unwired: 1 in, 2 out]
          }
        }
      }
      frame "Stop roller" {
        n455 = local read "Connected?"() -> (w819:bool)
        n456 = case shown="True" w819 {
          tunnel: [w821 w827] -> w816
          tunnel: w817 -> [w821 w825]
          tunnel: w818 -> [_ w824]
          frame False {
            # "Don't bother trying to send a message to the RT system if UI Main VI isn't even connected"
          }
          frame True {
            n457 = global read "Global - UI Stream and Variable Connections.vi" "UI Command Stream"() -> (w823:refnum<k21>)
            n458 = Bundle("Message"="Update Manual Values", "Message Data"=w824) -> (w826:T16)  [unwired: 1 in]
            n459 = shared-variable-write(w823, w825, w826) -> (w827:errorcluster)  [unwired: 1 in, 2 out]
          }
        }
      }
      frame "Home stage" {
        n460 = local read "Connected?"() -> (w829:bool)
        n461 = case shown="True" w829 {
          tunnel: w831 -> [w833 w839]
          tunnel: [w833 w838] -> w830
          tunnel: w828 -> [_ w834]
          frame False {
            # "Don't bother trying to send a message to the RT system if UI Main VI isn't even connected"
          }
          frame True {
            n462 = global read "Global - UI Stream and Variable Connections.vi" "UI Command Stream"() -> (w835:refnum<k21>)
            n463 = Bundle("Home stage", "Message Data"=w834) -> (w836:cluster{string, "Message Data":variant})  [unwired: 1 in]
            n464 = shared-variable-write(w835, w839, w836) -> (w838:errorcluster)  [unwired: 1 in, 2 out]
          }
        }
      }
      frame "Go stage" {
        n465 = local read "Connected?"() -> (w841:bool)
        n466 = case shown="True" w841 {
          tunnel: w843 -> [w845 w851]
          tunnel: [w845 w850] -> w842
          tunnel: w840 -> [_ w846]
          frame False {
            # "Don't bother trying to send a message to the RT system if UI Main VI isn't even connected"
          }
          frame True {
            n467 = global read "Global - UI Stream and Variable Connections.vi" "UI Command Stream"() -> (w847:refnum<k21>)
            n468 = Bundle("Go stage", "Message Data"=w846) -> (w848:cluster{string, "Message Data":variant})  [unwired: 1 in]
            n469 = shared-variable-write(w847, w851, w848) -> (w850:errorcluster)  [unwired: 1 in, 2 out]
          }
        }
      }
      frame "Stop stage" {
        n470 = local read "Connected?"() -> (w852:bool)
        n471 = case shown="True" w852 {
          tunnel: w854 -> [w857 w863]
          tunnel: [w857 w862] -> w855
          tunnel: w853 -> [_ w858]
          frame False {
            # "Don't bother trying to send a message to the RT system if UI Main VI isn't even connected"
          }
          frame True {
            n472 = global read "Global - UI Stream and Variable Connections.vi" "UI Command Stream"() -> (w859:refnum<k21>)
            n473 = Bundle("Stop stage", "Message Data"=w858) -> (w860:cluster{string, "Message Data":variant})  [unwired: 1 in]
            n474 = shared-variable-write(w859, w863, w860) -> (w862:errorcluster)  [unwired: 1 in, 2 out]
          }
        }
      }
      frame "Exit" {
        # "Close all connections"
        # "Stop Monitoring Loop"
        # "Stop Event Handling Loop"
        # "Release the UI Message queue reference"
        # "Stop UI Message Loop"
        # "Exit - Fire the User Event to stop the Event Handling Loop, and toggle the local variable to stop the Monitoring Loop.  This message alone causes all three loops to stop."
        n475 = global write "Global - All UI Loop Stop.vi" "All UI Loop Stop"(TRUE ("Stop Monitoring Loop")) -> ()
        n476 = call "Fire User Event - Stop.vi"("User Event - Stop"=w872) -> ("error out"=w871:errorcluster)  [unwired: 10 in]
        n477 = Release Queue(queue=w868, error in (no error)=w873) -> (error out=w869:errorcluster)  [unwired: 1 in, 2 out]
        n478 = global read "Global - UI Stream and Variable Connections.vi" "UI Command Stream"() -> (w866:refnum<k21>)
        n479 = global read "Global - UI Stream and Variable Connections.vi" "RT Message Stream"() -> (w865:refnum<k21>)
        n480 = global read "Global - UI Stream and Variable Connections.vi" "Variable References"() -> (w864:T10)
        n481 = Destroy Stream Endpoint(11:w866) -> ()  [unwired: 1 in, 1 out]
        n482 = Destroy Stream Endpoint(11:w865) -> ()  [unwired: 1 in, 1 out]
        n483 = call "Close Variable Connections.vi"("Variable References"=w864) -> ()  [unwired: 11 in]
        n484 = Merge Errors(w871, w869) -> (w874:errorcluster)
      }
      frame "---Copy This Frame---" {
        # "Duplicate this frame when creating new messages.  Change this comment in the duplicated frame to describe this message."
        n485 = Merge Errors(w878) -> (w877:errorcluster)
      }
      frame Default {
        # "'Default' case only runs if there is a message that isn't defined in any of the other cases.  Output a programming error."
        n486 = Format Into String(format string="The invalid message string \"%s\" was received in the Message Handling Loop." ("Invalid Message Loop Message"), w883) -> (resulting string=w880:string)  [unwired: 2 in, 1 out]
        n487 = call <vilib>:"Error Cluster From Error Code.vi"("error message (\"\")"=w880, "error code (0)"=1) -> ("error out"=w881:errorcluster)  [unwired: 7 in]
      }
    }
    n488 = call "UI Error Handler - Message Handler.vi"("error in (no error)"=w460, "Message Queue"=w461) -> ()  [unwired: 9 in, 1 out]
    n489 = call <vilib>:"Clear Errors.vi"("error in (no error)"=w460) -> ("error out"=w459:errorcluster)  [unwired: 6 in]
  }
  n490 = while {
    tunnel: w11 -> [w907]
    shift-right: [w900] -> _
    shift-left: dbl[] [] -> [w899]
    shift-right: [w898] -> _
    shift-left: dbl[] [] -> [w895]
    shift-right: [w897] -> _
    shift-left: dbl[] [] -> [w896]
    shift-right: [w894] -> _
    shift-left: dbl[] [] -> [w891]
    shift-right: [w893] -> _
    shift-left: dbl[] [] -> [w890]
    shift-right: [w892] -> _
    shift-left: dbl[] [] -> [w889]
    shift-right: [w886] -> _
    shift-left: dbl[] [] -> [w887]
    stop <- w908 stop-if-true
    (unwired) refnum<vi> refnum ("Controller Calculations")
    # "Only read monitoring variables if:\n1.The UI Main VI is \nconnected to the RT target\nAND\n2. The Pause button is not depressed\nAND\n3. The Save button is not depressed"
    # "Only the 'Exit' message in the UI Message Loop can stop the Monitoring Loop."
    # "Monitoring Loop"
    n491 = local read "Connected?"() -> (w905:bool)
    n492 = Not(x="Pause Button") -> (.not. x?=w902:bool)
    n493 = Divide(x=1000.0, y="Display frequency (Hz)") -> (x/y=w888:dbl)
    n494 = To Unsigned Long Integer(number=w888) -> (unsigned 32bit integer=w885:u32)
    n495 = global write "Global - Configuration Options.vi" "Monitoring Loop Rate (ms)"(w885) -> ()
    n496 = And(x=w905, y=w902) -> (x .and. y?=w903:bool)
    n497 = case shown="True" w903 {
      tunnel: w907 -> [_ w1052]
      tunnel: w888 -> [w925 w1047]
      tunnel: [w923 w991] -> w900
      tunnel: w899 -> [w922 w1042]
      tunnel: [w918 w989] -> w898
      tunnel: [w920 w990] -> w897
      tunnel: w896 -> [w921 w1036]
      tunnel: w895 -> [w919 w1035]
      tunnel: [w916 w988] -> w894
      tunnel: [w914 w987] -> w893
      tunnel: [w912 w986] -> w892
      tunnel: w891 -> [w917 w1028]
      tunnel: w890 -> [w915 w1027]
      tunnel: w889 -> [w913 w1026]
      tunnel: w888 -> [_ w1018]
      tunnel: w887 -> [w911 w973]
      tunnel: [w910 w968] -> w886
      frame False {
        n498 = local read "Clear Button"() -> (w909:bool)
        n499 = Wait (ms)(milliseconds to wait=w925) -> ()  [unwired: 1 out]
        n500 = Not(x=w909) -> (.not. x?=w924:bool)
        n501 = case shown="False" w924 {
          tunnel: [w939 w954] -> w923
          tunnel: w922 -> [w938 w954]
          tunnel: w921 -> [w937 w953]
          tunnel: [w936 w953] -> w920
          tunnel: w919 -> [w935 w952]
          tunnel: [w934 w952] -> w918
          tunnel: w917 -> [w933 w951]
          tunnel: [w932 w951] -> w916
          tunnel: w915 -> [w931 w950]
          tunnel: [w930 w950] -> w914
          tunnel: w913 -> [w929 w949]
          tunnel: [w928 w949] -> w912
          tunnel: w911 -> [w927 w948]
          tunnel: [w926 w948] -> w910
          frame False {
            n502 = stacked-sequence {
              tunnel: [dbl[] [] _] -> w939
              tunnel: w938 -> [_ _]
              tunnel: w937 -> [_ _]
              tunnel: [dbl[] [] _] -> w936
              tunnel: w935 -> [_ _]
              tunnel: [dbl[] [] _] -> w934
              tunnel: w933 -> [_ _]
              tunnel: [dbl[] [] _] -> w932
              tunnel: w931 -> [_ _]
              tunnel: [dbl[] [] _] -> w930
              tunnel: w929 -> [_ _]
              tunnel: [dbl[] [] _] -> w928
              tunnel: w927 -> [_ _]
              tunnel: [dbl[] [] _] -> w926
              frame #0 {
                # "Clear all arrays"
              }
              frame #1 {
                w947 = FALSE ("Clear Button")
                n503 = local write "Pause Button"(w947) -> ()
                n504 = local write "Clear Button"(w947) -> ()
              }
            }
          }
          frame True {
          }
        }
      }
      frame True {
        # "Build the array for plotting"
        # "Get the time data"
        # "Serialize the shared variable calls to simplify the scheduling performed by LabVIEW at runtime"
        n505 = global read "Global - UI Stream and Variable Connections.vi" "Variable References"() -> (w1050:T10)
        n506 = call "UI - Read Stream from RT.vi"("Message Queue"=w1052) -> ("error out"=w1058:errorcluster, "Message Received?"=w1048:bool, "dup Message Queue"=w1051:refnum<queue>)  [unwired: 8 in]
        n507 = case shown="False" w1048 {
          tunnel: w1047 -> [w1118 _]
          frame False {
            n508 = Wait (ms)(milliseconds to wait=w1118) -> ()  [unwired: 1 out]
          }
          frame True {
            # "If a message was received, immediately read again"
          }
        }
        n509 = Unbundle By Name(w1050) -> ("CPU Usage"=w1064:refnum<k21>, "Contiguous Memory"=w1063:refnum<k21>, "Input Values"=w1062:refnum<k21>, "Output Values"=w1061:refnum<k21>, "FPGA Mode"=w1060:refnum<k21>, "Actual Loop Period"=w1059:refnum<k21>)
        n510 = Divide(x=w1018, y=2.0) -> (x/y=w974:dbl)
        n511 = shared-variable-read(w1064, w1058) -> (w1057:errorcluster, →"CPU Usage (%)":dbl)  [unwired: 2 out]
        n512 = shared-variable-read(w1063, w1057) -> (w1056:errorcluster, →"Largest Contiguous Memory (bytes)":dbl)  [unwired: 2 out]
        n513 = shared-variable-read(w1062, w1056) -> (w1055:errorcluster, w1066:T11)  [unwired: 2 out]
        n514 = shared-variable-read(w1061, w1055) -> (w1054:errorcluster, w1065:T11)  [unwired: 2 out]
        n515 = shared-variable-read(w1060, w1054) -> (w1053:errorcluster, →"Current FPGA Control Mode":T18)  [unwired: 2 out]
        n516 = shared-variable-read(w1059, w1053) -> (w955:errorcluster, w1017:u32)  [unwired: 2 out]
        "Actual Loop Period (ticks)" <- w1017
        n517 = To Double Precision Float(number=w1066) -> (double precision float=w1046:T12)
        n518 = To Double Precision Float(number=w1065) -> (double precision float=w1069:T12)
        n519 = shared-variable "NI-cRIO9075-01756F19\\Shared Variables.lvlib\\Stage position"() -> (w979:dbl)  [unwired: 1 in, 1 out]
        "Stage position (mm):" <- w979
        n520 = Unbundle By Name(w1069) -> ("Channel 0"=w1034:dbl, "Channel 1"=w981:dbl, "Channel 2"=w980:dbl)
        n521 = Unbundle By Name(w1046) -> ("Channel 0"=w1023:dbl, "Channel 1"=w1039:dbl)
        n522 = Get Date/Time In Seconds() -> (seconds since 1Jan1904=w1043:timestamp)
        n523 = Multiply(x=1000.0, y=w1023) -> (x*y=w1022:dbl)
        n524 = To Double Precision Float(number=w1043) -> (double precision float=w1025:dbl)
        n525 = Build Array(w1022) -> (w1037:dbl[])
        n526 = Build Array(w1039) -> (w1038:dbl[])
        n527 = Build Array(w1034) -> (w1033:dbl[])
        n528 = Build Array(w981) -> (w1032:dbl[])
        n529 = Build Array(w980) -> (w1031:dbl[])
        n530 = Build Array(w979) -> (w978:dbl[])
        n531 = Build Array (concatenate)(w1042, w1025) -> (w997:dbl[])
        n532 = Build Array (concatenate)(w1036, w1037) -> (w1001:dbl[])
        n533 = Build Array (concatenate)(w1035, w1038) -> (w1004:dbl[])
        n534 = Build Array (concatenate)(w1028, w1033) -> (w1007:dbl[])
        n535 = Build Array (concatenate)(w1027, w1032) -> (w1010:dbl[])
        n536 = Build Array (concatenate)(w1026, w1031) -> (w1013:dbl[])
        n537 = Build Array (concatenate)(w973, w978) -> (w977:dbl[])
        n538 = Divide(x=u32 40000000, y=w1017) -> (x/y=→"Control loop frequency (Hz)":dbl)
        n539 = call "Convert to Dynamic Data2"("Array"=w1004) -> ("Dynamic Data Type"=w1003:dynamicdata)  [unwired: 3 in]
        n540 = call "Convert to Dynamic Data6"("Array"=w1013) -> ("Dynamic Data Type"=w1012:dynamicdata)  [unwired: 3 in]
        n541 = call "Convert to Dynamic Data3"("Array"=w1007) -> ("Dynamic Data Type"=w1006:dynamicdata)  [unwired: 3 in]
        n542 = call "Convert to Dynamic Data4"("Array"=w1010) -> ("Dynamic Data Type"=w1009:dynamicdata)  [unwired: 3 in]
        n543 = call "Convert to Dynamic Data"("Array"=w1001) -> ("Dynamic Data Type"=w1000:dynamicdata)  [unwired: 3 in]
        n544 = call "Convert to Dynamic Data5"("Array"=w977) -> ("Dynamic Data Type"=w976:dynamicdata)  [unwired: 3 in]
        n545 = call "Filter"("Lower Cut-Off"=w974, "Signal"=w1003) -> ("Filtered Signal"=w1002:dynamicdata)  [unwired: 8 in, 1 out]
        n546 = call "Filter"("Lower Cut-Off"=w974, "Signal"=w1012) -> ("Filtered Signal"=w1011:dynamicdata)  [unwired: 8 in, 1 out]
        n547 = call "Filter"("Lower Cut-Off"=w974, "Signal"=w1006) -> ("Filtered Signal"=w1005:dynamicdata)  [unwired: 8 in, 1 out]
        n548 = call "Filter"("Lower Cut-Off"=w974, "Signal"=w1009) -> ("Filtered Signal"=w1008:dynamicdata)  [unwired: 8 in, 1 out]
        n549 = call "Filter"("Lower Cut-Off"=w974, "Signal"=w1000) -> ("Filtered Signal"=w999:dynamicdata)  [unwired: 8 in, 1 out]
        n550 = call "Filter2"("Lower Cut-Off"=w974, "Signal"=w976) -> ("Filtered Signal"=w975:dynamicdata)  [unwired: 8 in, 1 out]
        n551 = call "Convert from Dynamic Data2"("Dynamic Data Type"=w1002) -> ("Array"=w995:dbl[])  [unwired: 3 in]
        n552 = call "Convert from Dynamic Data6"("Dynamic Data Type"=w1011) -> ("Array"=w992:dbl[])  [unwired: 3 in]
        n553 = call "Convert from Dynamic Data3"("Dynamic Data Type"=w1005) -> ("Array"=w994:dbl[])  [unwired: 3 in]
        n554 = call "Convert from Dynamic Data4"("Dynamic Data Type"=w1008) -> ("Array"=w993:dbl[])  [unwired: 3 in]
        n555 = call "Convert from Dynamic Data"("Dynamic Data Type"=w999) -> ("Array"=w996:dbl[])  [unwired: 3 in]
        n556 = call "Convert from Dynamic Data5"("Dynamic Data Type"=w975) -> ("Array"=w970:dbl[])  [unwired: 3 in]
        n557 = Array Size(array=w997) -> (size(s)=w1044:i32)
        n558 = Greater?(x=w1044, y="Number of points") -> (0:w1045:bool)
        n559 = case shown="True" w1045 {
          tunnel: w996 -> [w1099 w1114]
          tunnel: w997 -> [w1100 w1116]
          tunnel: w1044 -> [_ w1117]
          tunnel: "Number of points" -> [_ w1103]
          tunnel: [w1100 w1115] -> w972
          tunnel: [w1099 w1113] -> w985
          tunnel: w995 -> [w1098 w1111]
          tunnel: [w1098 w1112] -> w984
          tunnel: [w1095 w1110] -> w983
          tunnel: [w1097 w1109] -> w961
          tunnel: [w1096 w1108] -> w965
          tunnel: w994 -> [w1095 w1107]
          tunnel: w993 -> [w1097 w1106]
          tunnel: w992 -> [w1096 w1105]
          tunnel: w970 -> [w1094 w1102]
          tunnel: [w1094 w1101] -> w969
          frame False {
          }
          frame True {
            n560 = Subtract(x=w1117, y=w1103) -> (x-y=w1104:i32)
            n561 = Array Subset(array=w1116, index=w1104, length=w1103) -> (w1115:dbl[])
            n562 = Array Subset(array=w1114, index=w1104, length=w1103) -> (w1113:dbl[])
            n563 = Array Subset(array=w1111, index=w1104, length=w1103) -> (w1112:dbl[])
            n564 = Array Subset(array=w1107, index=w1104, length=w1103) -> (w1110:dbl[])
            n565 = Array Subset(array=w1106, index=w1104, length=w1103) -> (w1109:dbl[])
            n566 = Array Subset(array=w1105, index=w1104, length=w1103) -> (w1108:dbl[])
            n567 = Array Subset(array=w1102, index=w1104, length=w1103) -> (w1101:dbl[])
          }
        }
        n568 = case shown="False" "Retain data" {
          tunnel: w997 -> [_ w1093]
          tunnel: w996 -> [_ w1092]
          tunnel: w995 -> [_ w1091]
          tunnel: w994 -> [_ w1090]
          tunnel: w993 -> [_ w1089]
          tunnel: w992 -> [_ w1088]
          tunnel: [w1081 w1093] -> w991
          tunnel: [w1082 w1092] -> w990
          tunnel: [w1083 w1091] -> w989
          tunnel: [w1084 w1090] -> w988
          tunnel: [w1085 w1089] -> w987
          tunnel: [w1086 w1088] -> w986
          tunnel: w972 -> [w1081 _]
          tunnel: w985 -> [w1082 _]
          tunnel: w984 -> [w1083 _]
          tunnel: w983 -> [w1084 _]
          tunnel: w961 -> [w1085 _]
          tunnel: w965 -> [w1086 _]
          tunnel: w970 -> [_ w1087]
          tunnel: [w1080 w1087] -> w968
          tunnel: w969 -> [w1080 _]
          frame False {
          }
          frame True {
          }
        }
        n569 = call <vilib>:"Std Deviation and Variance.vi"("X"=w961) -> ("mean"=→"F avg":dbl, "standard deviation"=→"F std":dbl)  [unwired: 1 in, 1 out]
        n570 = Array Size(array=w965) -> (size(s)=w966:i32)
        n571 = Bundle(w972, "Array"=w985) -> (w1041:cluster{dbl[], "Array":dbl[]})  [unwired: 1 in]
        n572 = Bundle(w972, "Array"=w984) -> (w1040:cluster{dbl[], "Array":dbl[]})  [unwired: 1 in]
        n573 = Bundle(w972, "Array"=w961) -> (w956:cluster{dbl[], "Array":dbl[]})  [unwired: 1 in]
        "Force (N)" <- w956
        n574 = Bundle(w972, "Array"=w983) -> (→"V*":cluster{dbl[], "Array":dbl[]})  [unwired: 1 in]
        n575 = Bundle(w972, "Array"=w965) -> (→"Roller position (mm)":cluster{dbl[], "Array":dbl[]})  [unwired: 1 in]
        n576 = Bundle(w972, "Array"=w969) -> (→"Stage position (mm)":cluster{dbl[], "Array":dbl[]})  [unwired: 1 in]
        n577 = Decrement(x=w966) -> (x-1=w967:i32)
        n578 = Build Array(w1041, w1040) -> (→"Inputs (mV or V)":cluster{dbl[], "Array":dbl[]}[])
        n579 = Index Array(array=w965, index=w967) -> (element=w964:dbl)
        n580 = Array Size(array=w961) -> (size(s)=w962:i32)
        n581 = Decrement(x=w962) -> (x-1=w963:i32)
        n582 = local read "Roller LED"() -> (w960:bool)
        n583 = Index Array(array=w961, index=w963) -> (element=w957:dbl)
        n584 = local read "Roller LED"() -> (w959:bool)
        n585 = local read "Test LED"() -> (w958:bool)
        n586 = case shown="True" w958 {
          tunnel: w957 -> [_ w1075]
          tunnel: w956 -> [_ w1074]
          frame False {
            n587 = local write "Measured contact force (N):"(0.0 ("Measured contact force (N):")) -> ()
            n588 = local write "Stage position (mm):"(0.0 ("Stage position (mm):")) -> ()
            n589 = local write "Force results (N)"(cluster{dbl[], dbl[]} {array[1000 elements], array[1000 elements]} ("Force results (N)")) -> ()
          }
          frame True {
            n590 = shared-variable "NI-cRIO9075-01756F19\\Shared Variables.lvlib\\Stage position"() -> (→"Stage position (mm):":dbl)  [unwired: 1 in, 1 out]
            "Measured contact force (N):" <- w1075
            "Force results (N)" <- w1074
          }
        }
        n591 = case shown="True" w960 {
          tunnel: w964 -> [_ w1079]
          frame False {
            n592 = local write "Position (mm):"(0.0 ("Position (mm):")) -> ()
          }
          frame True {
            "Position (mm):" <- w1079
          }
        }
        n593 = case shown="True" w959 {
          tunnel: w957 -> [_ w1077]
          frame False {
            n594 = local write "Force (N):"(0.0 ("Force (N):")) -> ()
          }
          frame True {
            "Force (N):" <- w1077
          }
        }
        n595 = call "UI Error Handler - Monitoring.vi"("error in (no error)"=w955, "Message Queue"=w1051) -> ()  [unwired: 9 in, 1 out]
      }
    }
    n596 = global read "Global - All UI Loop Stop.vi" "All UI Loop Stop"() -> (w908:bool)
  }
  n597 = Unregister For Events(event registration refnum=w14, error in=w22) -> (error out=w15:errorcluster)
  n598 = Merge Errors(w15, w23) -> (w21:errorcluster)
  n599 = call "Destroy User Event - Stop.vi"("error in (no error)"=w21, "User Event - Stop"=w19) -> ("error out"=w12:errorcluster)  [unwired: 9 in]
  n600 = call <vilib>:"Simple Error Handler.vi"("error in (no error)"=w12) -> ()  [unwired: 4 in, 5 out]
  "Max position (mm):" <- 151.49760546875
  "Max speed (mm/s):" <- 21.0 ("Max speed (mm/s):")
